vi "adsorption_rig_main-automation.vi"() -> ()   [LabVIEW 2024]
uses:
  adam5000_LLB/controls/adam-5000-serial-settings.ctl
  adam5000_LLB/controls/adam-5000-cmd-response.ctl
  adam5000_LLB/controls/state-enum.ctl
  adam5000_LLB/sub-vi/csv-file-logging/filepath-selection.ctl
  controls/sequence-states.ctl
  adam5000_LLB/controls/adam-5000-all-chassis-data.ctl
  adam5000_LLB/controls/adam-5000-all-module-datas.ctl
  adam5000_LLB/controls/digital-output-cluster.ctl
  adam5000_LLB/controls/digitial-input-cluster.ctl
  adam5000_LLB/controls/analog-output-cluster.ctl
  adam5000_LLB/controls/analog-input-cluster.ctl
  adam5000_LLB/controls/thermocouple-input-cluster.ctl
  adam5000_LLB/controls/adam-5000-chassis-cmd-ack.ctl
  adam5000_LLB/controls/adam-5000-chassis-module-types.ctl
  adam5000_LLB/controls/adam-5000-DO-user-input.ctl
  adam5000_LLB/controls/adam-5000-status-indicator-references.ctl
  controls/sequence-timings.ctl
  controls/state-indicator.ctl
panel:
  in  "Reset LD":bool
  out "longest delay":u32
  out "Next Log Event mS":u32
  in  "Tab Control":enum32{"System", "Settings"}(tab)
  out "Cycles Complete":u16
  out "sequence-state":T1
  out "pre":bool
  in  "Stop Sequence":bool
  in  "Start Sequence":bool
  out "Recirc":bool
  out "HR B":bool
  out "Ads 2":bool
  out "TC5":dbl
  out "TC1":dbl
  out "TC4":dbl
  in  "HR_B Time (s)":dbl
  in  "Ads_2 Time (s)":dbl
  in  "Isos_2 Time (s)":dbl
  out "Isos 2":bool
  out "HR A":bool
  out "Ads 1":bool
  out "TC12":dbl
  out "Isos 1":bool
  in  "# Cycles":u16=1
  in  "Recirc Time (s)":dbl
  in  "HR_A Time (s)":dbl
  in  "Ads_1 Time (s)":dbl
  in  "Isos_1 Time (s)":dbl
  in  "Flow 4":dbl
  in  "Flow 3":dbl
  in  "Flow 2":dbl
  in  "Flow 1":dbl
  in  "V9: EP1":bool
  in  "V12: EP4":bool
  in  "V10: EP2":bool
  in  "V11: EP3":bool
  in  "V15: \nRecirculation":bool
  in  "V14: HR2":bool
  out "TC9":dbl
  in  "V13: HR1":bool
  out "TC8":dbl
  in  "V8: In4":bool
  out "TC2":dbl
  out "TC3":dbl
  out "TC6":dbl
  out "TC7":dbl
  out "TC10":dbl
  out "TC11":dbl
  in  "V1: Ex1":bool
  in  "V2: Ex2":bool
  in  "V4: Ex4":bool
  in  "V5: In1":bool
  in  "V6: In2":bool
  in  "V7: In3":bool
  out "P1: Condenser":dbl
  out "P2: Adsorber 2":dbl
  out "P3: Adsorber 1":dbl
  out "P4: Evaporator":dbl
  in  "V3: Ex3":bool
  in  "Additional CSV Data Heading":string="Flow1,Flow2,Flow3,Flow4"
  in  "Chassis Settings":T2={"VISA resource name"="COM4", "baud rate (19200)"=19200, "Chassis ID"=1}
  in  "Log Filepath Selection":T3={"Log Filepath Source"=enum."Application Relative (Auto)", "Log File Path (Manual)"=path "C:/Users/iwheard/Documents/0000-labview/adam5000-generic-controller/data", "Log File Folder Name"="data", "log file name"="log", "Include Date in Filename"=TRUE, "Include Time in Filename"=TRUE}
  out "Log Filepath":path
  out "log start time":u32
  out "log-elapsed time":dbl format="%.2f"
  in  "CSV Data Headings":string="time (s),T1,T2,T3,T4,T5,T6,T7,T8,T9,T10,T11,T12,P1,P2,P3,P4, state"
  out "Logged Data String":string
  out "error":errorcluster
  out "Hz":dbl format="%_3g"
  in  "Sample Rate (Hz)":dbl=1.0 min=0.0001 max=4.0 format="%#_4g"
  out "File Open":bool
  out "Logging Active":bool
  out "Error Detected":bool
  in  "Reset":bool
  out "ADAM Connected":bool
  in  "Stop ADAM":bool
  in  "Start Logging":bool
  out "Program State":T4
  in  "Start ADAM":bool
  out "cmd-response":T6
  out "Status Indicators":T7
  in  "Debug Mode":bool
  out "Loop Time (mS)":u32
  out "Loop Counter":i32
  in  "exit":bool
  # "Adsorption Rig 2026"
  # "Built By: \nImogen Heard"
  # "Cold"
  # "Ambient"
  # "Hot"
  # "Pressure Sensors"
  # "NV-002"
  # "NV-001"
  # "NV-004"
  # "Flow 4"
  # "Flow 1"
  # "Flow 2"
  # "Sequence"
  # "NV-003"
  # "Flow 3"
  # "Condenser"
  # "Adsorber 1"
  # "Adsorber 2"
  # "Evaporator"
  # "Flow Meter Inputs"
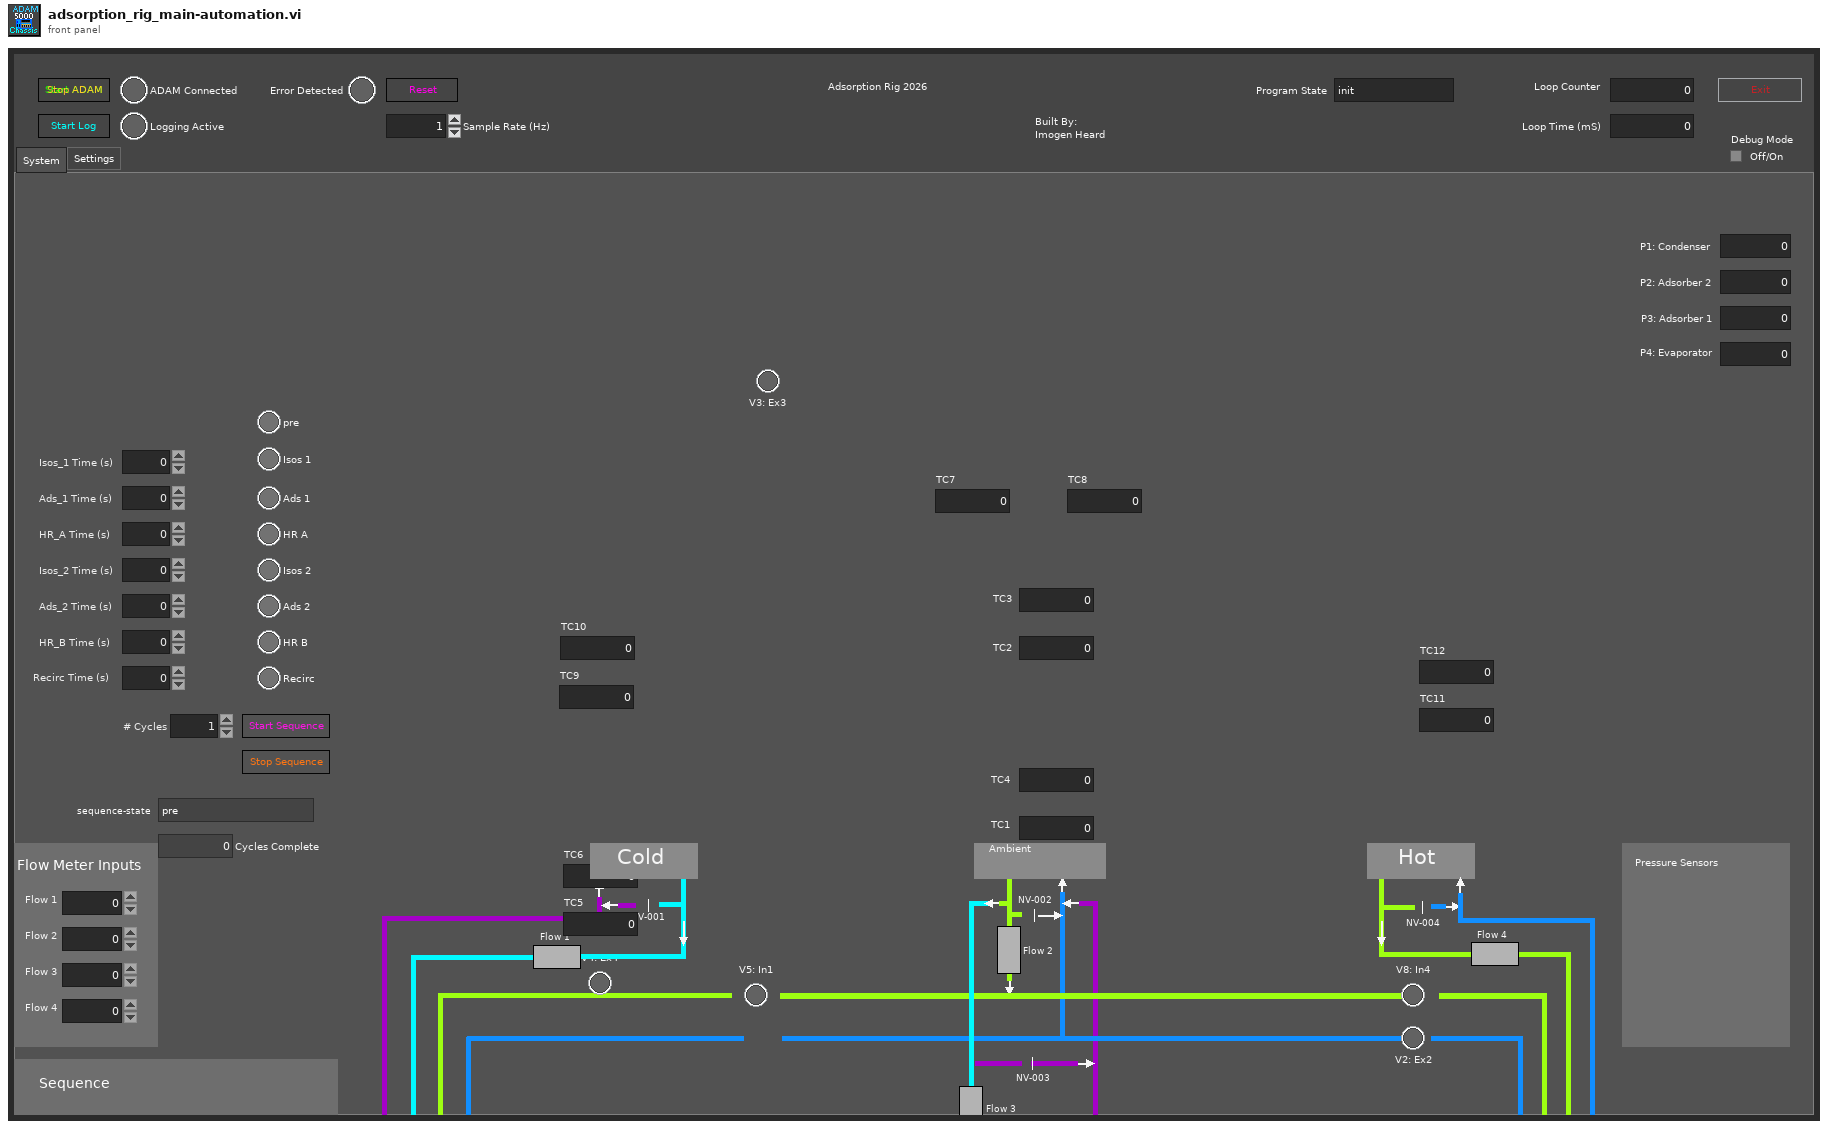
[diagram p1: front panel]
types:
  T1 = typedef "sequence-states.ctl" = enum16{"pre", "isos-1", "ads-1", "hr-a", "isos-2", "ads-2", "hr-b", "recirc", "cycle", "end"}
  T2 = typedef "adam-5000-serial-settings.ctl" = cluster{"VISA resource name":refnum<visa-resource-name>, "baud rate (19200)":u32, "Chassis ID":u8}
  T3 = typedef "filepath-selection.ctl" = cluster{"Log Filepath Source":enum16{"Application Relative (Auto)", "VI Relative (Auto)", "Complete Path (Manual)"}, "Log File Path (Manual)":path, "Log File Folder Name":string, "log file name":string, "Include Date in Filename":bool, "Include Time in Filename":bool}
  T4 = typedef "state-enum.ctl" = enum16{"init", "wait", "manual", "start", "run", "start-sequence", "stop-sequence", "sequence", "reset", "stop", "exit"}
  T5 = typedef "adam-5000-cmd-response.ctl" = cluster{"cmd string":string, "response":string}
  T6 = cluster{"cmd-response:0":T5, "cmd-response:1":T5, "cmd-response:2":T5, "cmd-response:3":T5, "cmd-response:4":T5, "cmd-response:5":T5, "cmd-response:6":T5, "cmd-response:7":T5}
  T7 = cluster{"status-indicator:0":cluster{"Sampling":bool, "Ack":bool}, "status-indicator:1":cluster{"Sampling":bool, "Ack":bool}, "status-indicator:2":cluster{"Sampling":bool, "Ack":bool}, "status-indicator:3":cluster{"Sampling":bool, "Ack":bool}, "status-indicator:4":cluster{"Sampling":bool, "Ack":bool}, "status-indicator:5":cluster{"Sampling":bool, "Ack":bool}, "status-indicator:6":cluster{"Sampling":bool, "Ack":bool}, "status-indicator:7":cluster{"Sampling":bool, "Ack":bool}}
  T8 = enum16{"Digital Output", "Digital Input", "Analog Output", "Analog Input", "Thermocouple", "Power Relay", "empty"}
  T9 = typedef "adam-5000-chassis-module-types.ctl" = cluster{"Slot 0: Module Type":enum16{"Digital Output", "Digital Input", "Analog Output", "Analog Input", "Thermocouple", "Power Relay", "empty"}, "Slot 1: Module Type":enum16{"Digital Output", "Digital Input", "Analog Output", "Analog Input", "Thermocouple", "Power Relay", "empty"}, "Slot 2: Module Type":enum16{"Digital Output", "Digital Input", "Analog Output", "Analog Input", "Thermocouple", "Power Relay", "empty"}, "Slot 3: Module Type":enum16{"Digital Output", "Digital Input", "Analog Output", "Analog Input", "Thermocouple", "Power Relay", "empty"}, "Slot 4: Module Type":enum16{"Digital Output", "Digital Input", "Analog Output", "Analog Input", "Thermocouple", "Power Relay", "empty"}, "Slot 5: Module Type":enum16{"Digital Output", "Digital Input", "Analog Output", "Analog Input", "Thermocouple", "Power Relay", "empty"}, "Slot 6: Module Type":enum16{"Digital Output", "Digital Input", "Analog Output", "Analog Input", "Thermocouple", "Power Relay", "empty"}, "Slot 7: Module Type":enum16{"Digital Output", "Digital Input", "Analog Output", "Analog Input", "Thermocouple", "Power Relay", "empty"}}
  T10 = typedef "adam-5000-chassis-cmd-ack.ctl" = cluster{"cmd-response:0":T5, "cmd-response:1":T5, "cmd-response:2":T5, "cmd-response:3":T5, "cmd-response:4":T5, "cmd-response:5":T5, "cmd-response:6":T5, "cmd-response:7":T5}
  T11 = typedef "adam-5000-all-chassis-data.ctl" = cluster{"slot:0":T12, "slot:1":T12, "slot:2":T12, "slot:3":T12, "slot:4":T12, "slot:5":T12, "slot:6":T12, "slot:7":T12}
  T12 = typedef "adam-5000-all-module-datas.ctl" = cluster{"Digital Outputs":T13, "Digital Inputs":T14, "Analog Outputs":T15, "Analog Inputs":T16, "Thermocouple Inputs (degC)":T17}
  T13 = typedef "digital-output-cluster.ctl" = cluster{"DO0":bool, "DO1":bool, "DO2":bool, "DO3":bool, "DO4":bool, "DO5":bool, "DO6":bool, "DO7":bool}
  T14 = typedef "digitial-input-cluster.ctl" = cluster{"DI0":bool, "DI1":bool, "DI2":bool, "DI3":bool, "DI4":bool, "DI5":bool, "DI6":bool, "DI7":bool}
  T15 = typedef "analog-output-cluster.ctl" = cluster{"AO0":dbl, "AO1":dbl, "AO2":dbl, "AO3":dbl}
  T16 = typedef "analog-input-cluster.ctl" = cluster{"AI0":dbl, "AI1":dbl, "AI2":dbl, "AI3":dbl, "AI4":dbl, "AI5":dbl, "AI6":dbl, "AI7":dbl}
  T17 = typedef "thermocouple-input-cluster.ctl" = cluster{"TC0":dbl, "TC1":dbl, "TC2":dbl, "TC3":dbl, "TC4":dbl, "TC5":dbl, "TC6":dbl}
  T18 = enum8{"Enabled", "Disabled", "Disabled and Grayed Out"}
  T19 = typedef "sequence-timings.ctl" = cluster{"Isos_1 Time":dbl, "Ads_1 Time":dbl, "HR_A Time":dbl, "Isos_2 Time":dbl, "Ads_2 Time":dbl, "HR_B Time":dbl, "Recirc Time":dbl}
  T20 = typedef "state-indicator.ctl" = cluster{"pre":bool, "Isos 1":bool, "Ads 1":bool, "HR A ":bool, "Isos 2":bool, "Ads 2":bool, "HR B":bool, "Recirc":bool}
  T21 = typedef "adam-5000-status-indicator-references.ctl" = cluster{"status-indicator:0":refnum<vi>, "status-indicator:1":refnum<vi>, "status-indicator:2":refnum<vi>, "status-indicator:3":refnum<vi>, "status-indicator:4":refnum<vi>, "status-indicator:5":refnum<vi>, "status-indicator:6":refnum<vi>, "status-indicator:7":refnum<vi>}
  T22 = typedef "adam-5000-DO-user-input.ctl" = cluster{"0:Digital Outputs":T13, "1:Digital Outputs":T13, "2:Digital Outputs":T13, "3:Digital Outputs":T13, "4:Digital Outputs":T13, "5:Digital Outputs":T13, "6:Digital Outputs":T13, "7:Digital Outputs":T13}
  T23 = cluster{"V1: Ex1":bool, "V2: Ex2":bool, "V3: Ex3":bool, "V4: Ex4":bool, "V5: In1":bool, "V6: In2":bool, "V7: In3":bool, "V8: In4":bool}
  T24 = cluster{"V9: EP1":bool, "V10: EP2":bool, "V11: EP3":bool, "V12: EP4":bool, "V13: HR1":bool, "V14: HR2":bool, "V15: \nRecirculation":bool, "V9: EP1":bool}
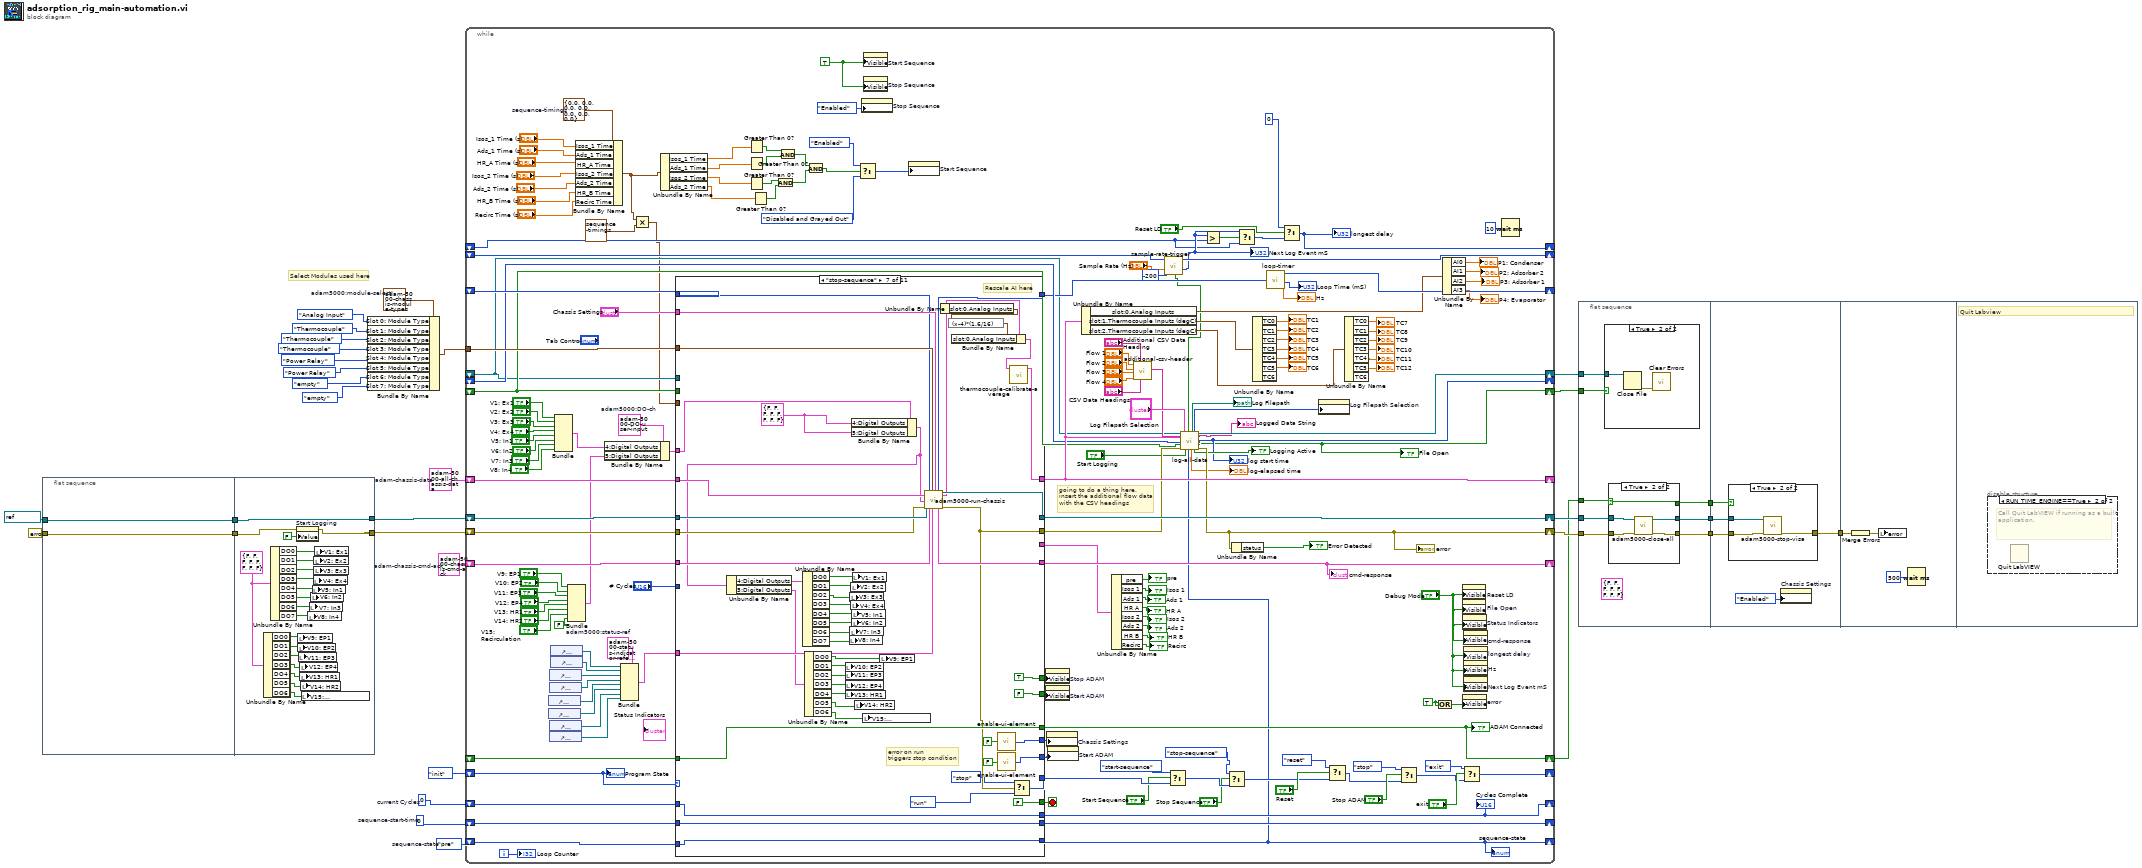
[diagram p0: block diagram]
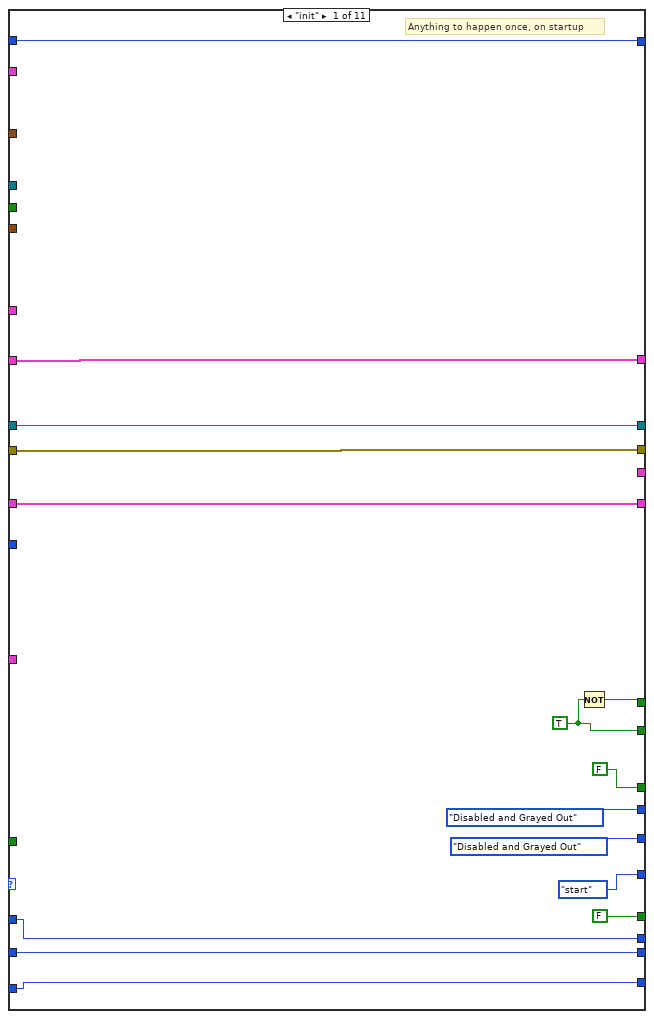
[diagram p6: hidden frame]
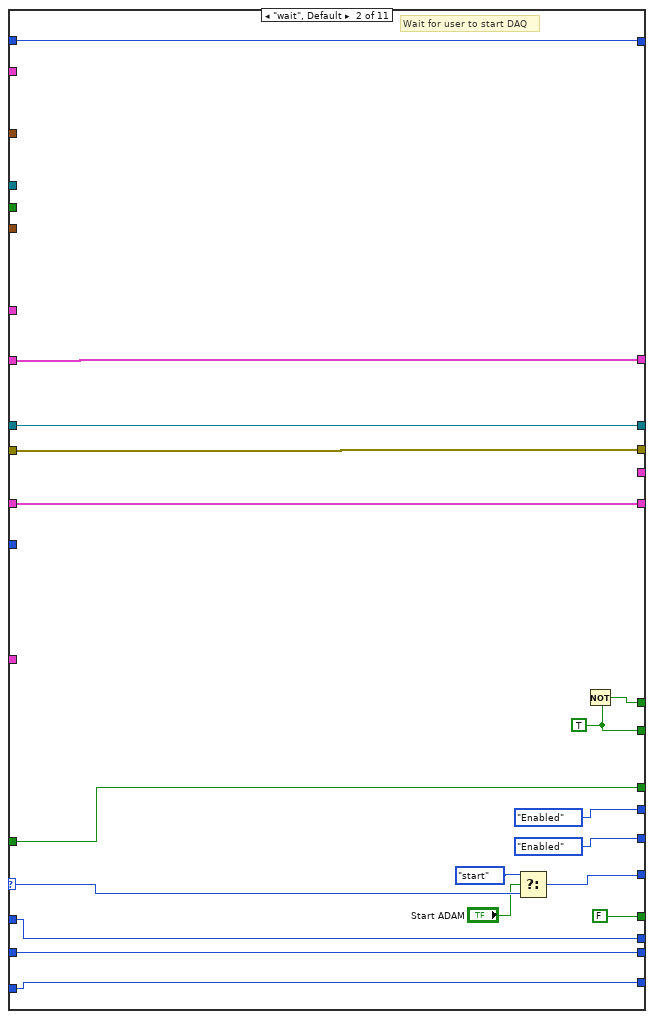
[diagram p7: hidden frame]
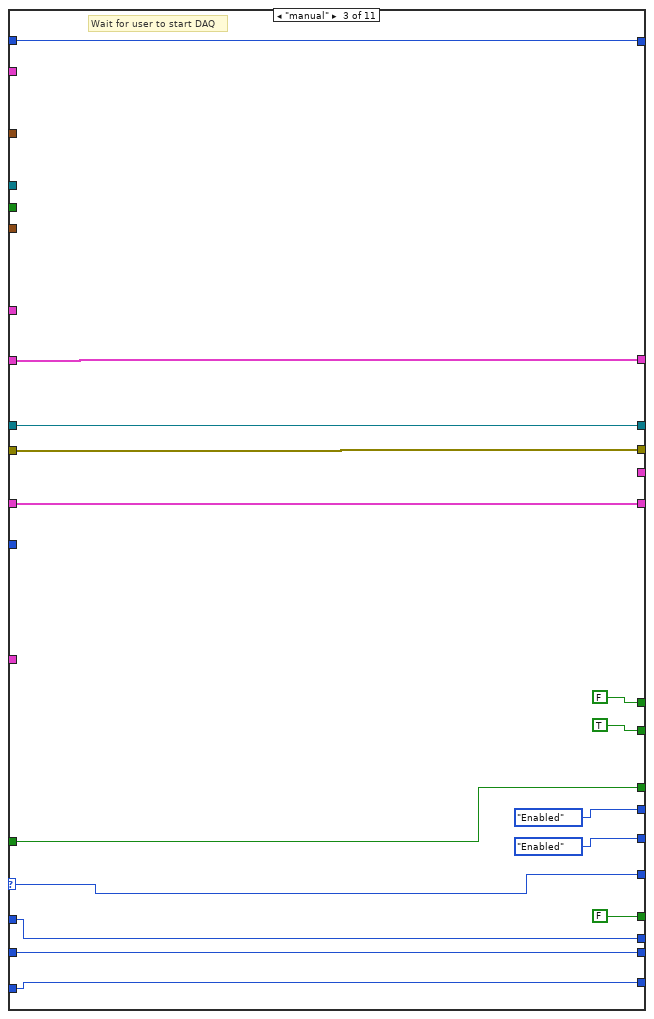
[diagram p8: hidden frame]
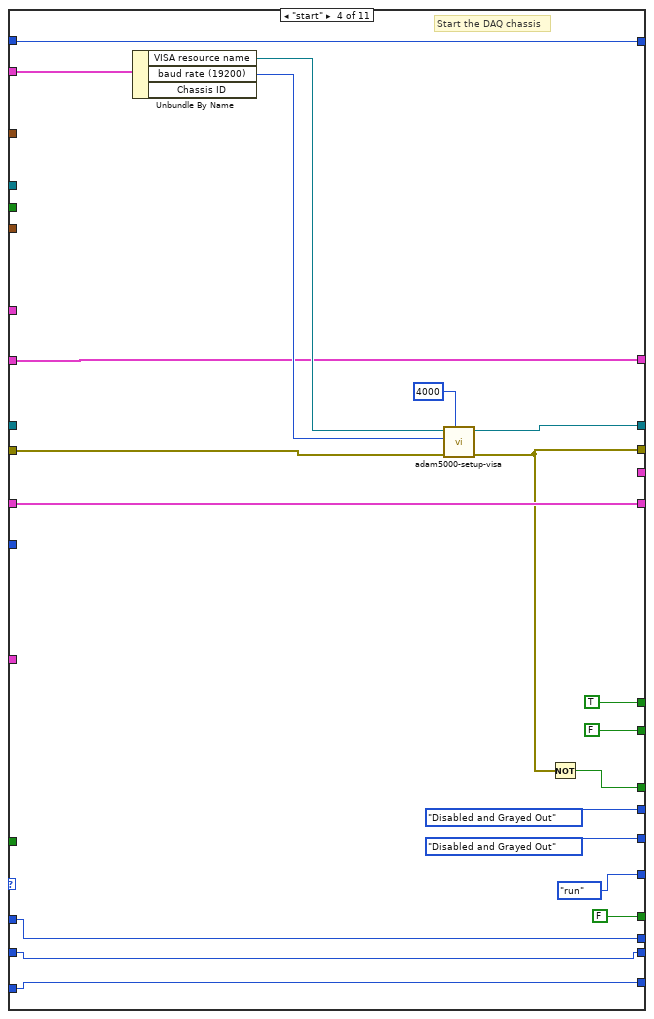
[diagram p9: hidden frame]
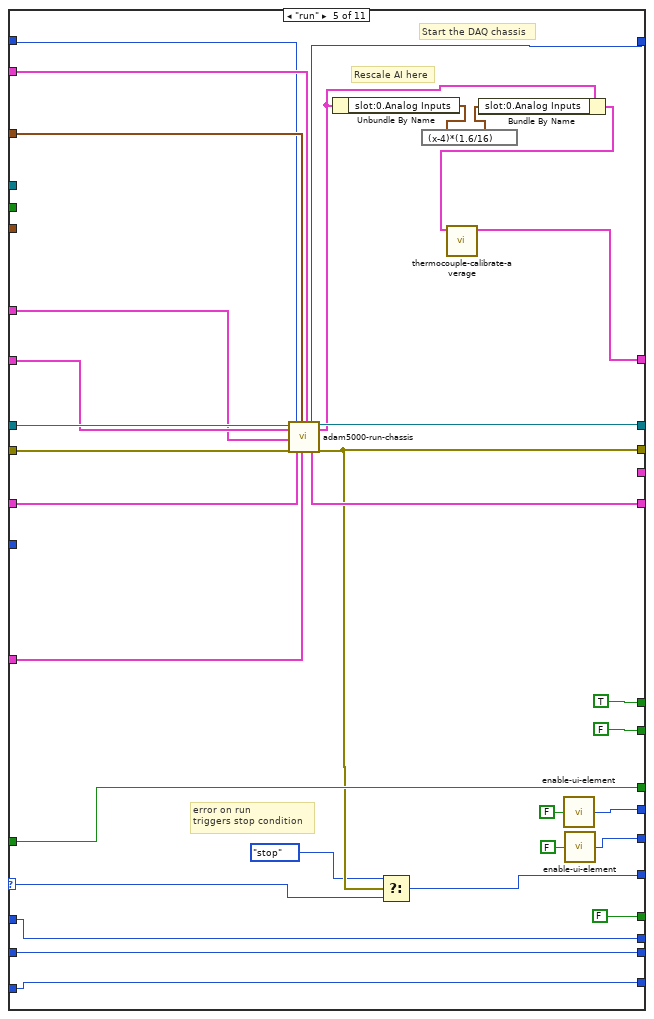
[diagram p10: hidden frame]
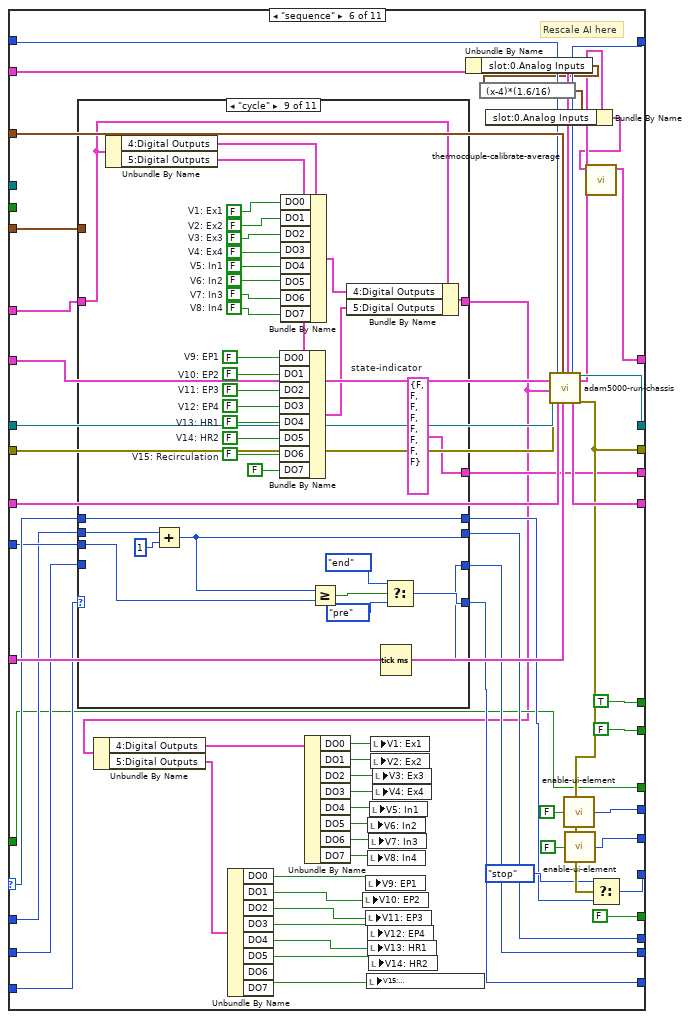
[diagram p11: hidden frame]
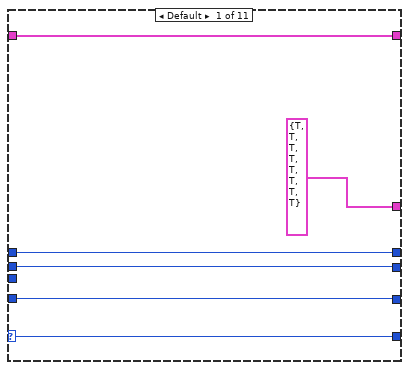
[diagram p12: hidden frame]
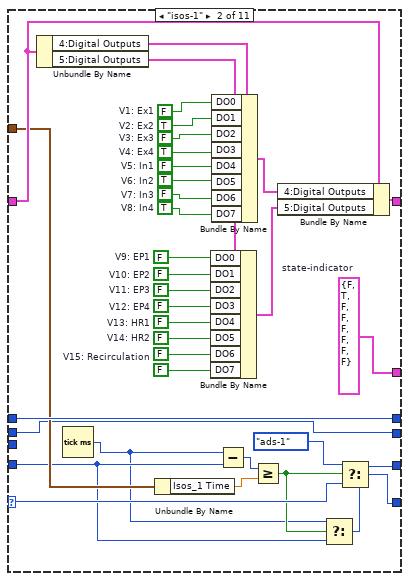
[diagram p13: hidden frame]
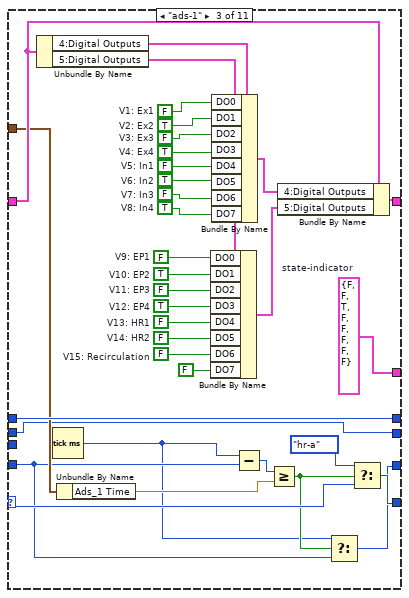
[diagram p14: hidden frame]
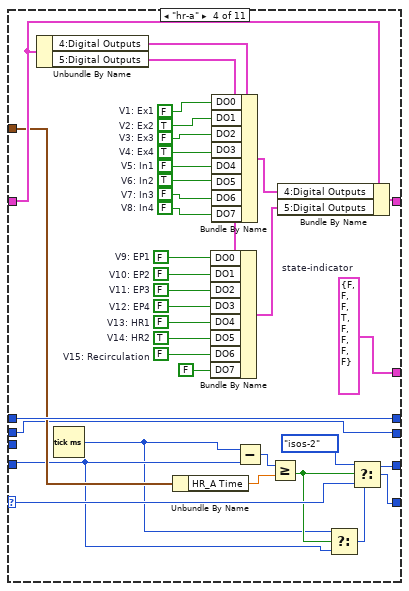
[diagram p15: hidden frame]
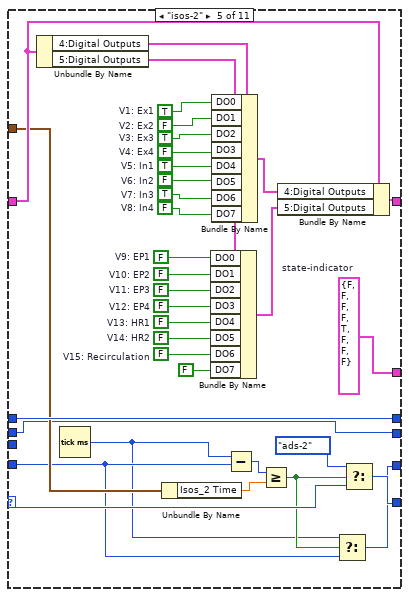
[diagram p16: hidden frame]
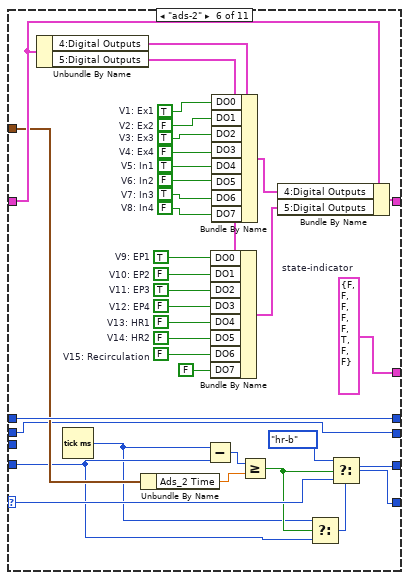
[diagram p17: hidden frame]
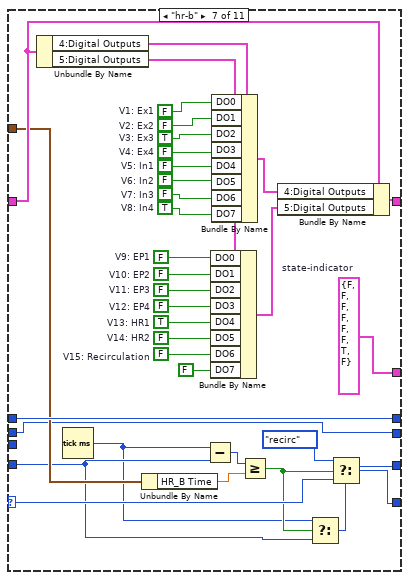
[diagram p18: hidden frame]
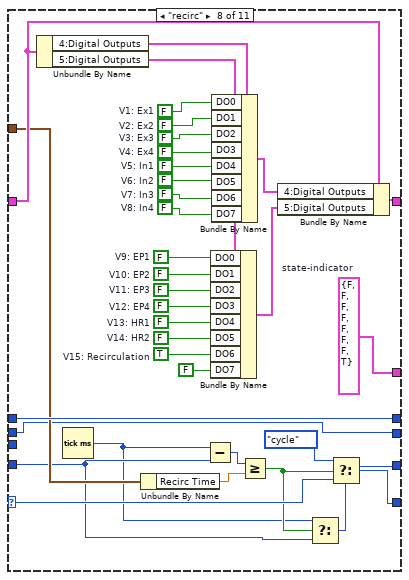
[diagram p19: hidden frame]
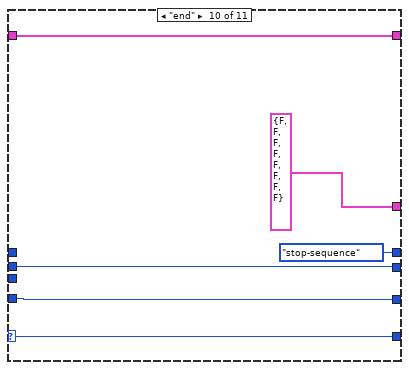
[diagram p20: hidden frame]
diagram:
  w1 = u16 0  # current Cycles
  w2 = u32 0  # sequence-start-time
  w3 = sequence-states."pre"  # sequence-state
  w23 = T9 {"Slot 0: Module Type"=enum."Digital Output", "Slot 1: Module Type"=enum."Digital Output", "Slot 2: Module Type"=enum."Digital Output", "Slot 3: Module Type"=enum."Digital Output", "Slot 4: Module Type"=enum."Digital Output", "Slot 5: Module Type"=enum."Digital Output", "Slot 6: Module Type"=enum."Digital Output", "Slot 7: Module Type"=enum."Digital Output"}  # adam5000:module-select
  w28 = T10 {"cmd-response:0"={"cmd string"="", "response"=""}, "cmd-response:1"={"cmd string"="", "response"=""}, "cmd-response:2"={"cmd string"="", "response"=""}, "cmd-response:3"={"cmd string"="", "response"=""}, "cmd-response:4"={"cmd string"="", "response"=""}, "cmd-response:5"={"cmd string"="", "response"=""}, "cmd-response:6"={"cmd string"="", "response"=""}, "cmd-response:7"={"cmd string"="", "response"=""}}  # adam-chassis-cmd-ack
  w29 = T11 {"slot:0"={"Digital Outputs"={"DO0"=FALSE, "DO1"=FALSE, "DO2"=FALSE, "DO3"=FALSE, "DO4"=FALSE, "DO5"=FALSE, "DO6"=FALSE, "DO7"=FALSE}, "Digital Inputs"={"DI0"=FALSE, "DI1"=FALSE, "DI2"=FALSE, "DI3"=FALSE, "DI4"=FALSE, "DI5"=FALSE, "DI6"=FALSE, "DI7"=FALSE}, "Analog Outputs"={"AO0"=0.0, "AO1"=0.0, "AO2"=0.0, "AO3"=0.0}, "Analog Inputs"={"AI0"=0.0, "AI1"=0.0, "AI2"=0.0, "AI3"=0.0, "AI4"=0.0, "AI5"=0.0, "AI6"=0.0, "AI7"=0.0}, "Thermocouple Inputs (degC)"={"TC0"=0.0, "TC1"=0.0, "TC2"=0.0, "TC3"=0.0, "TC4"=0.0, "TC5"=0.0, "TC6"=0.0}}, "slot:1"={"Digital Outputs"={"DO0"=FALSE, "DO1"=FALSE, "DO2"=FALSE, "DO3"=FALSE, "DO4"=FALSE, "DO5"=FALSE, "DO6"=FALSE, "DO7"=FALSE}, "Digital Inputs"={"DI0"=FALSE, "DI1"=FALSE, "DI2"=FALSE, "DI3"=FALSE, "DI4"=FALSE, "DI5"=FALSE, "DI6"=FALSE, "DI7"=FALSE}, "Analog Outputs"={"AO0"=0.0, "AO1"=0.0, "AO2"=0.0, "AO3"=0.0}, "Analog Inputs"={"AI0"=0.0, "AI1"=0.0, "AI2"=0.0, "AI3"=0.0, "AI4"=0.0, "AI5"=0.0, "AI6"=0.0, "AI7"=0.0}, "Thermocouple Inputs (degC)"={"TC0"=0.0, "TC1"=0.0, "TC2"=0.0, "TC3"=0.0, "TC4"=0.0, "TC5"=0.0, "TC6"=0.0}}, "slot:2"={"Digital Outputs"={"DO0"=FALSE, "DO1"=FALSE, "DO2"=FALSE, "DO3"=FALSE, "DO4"=FALSE, "DO5"=FALSE, "DO6"=FALSE, "DO7"=FALSE}, "Digital Inputs"={"DI0"=FALSE, "DI1"=FALSE, "DI2"=FALSE, "DI3"=FALSE, "DI4"=FALSE, "DI5"=FALSE, "DI6"=FALSE, "DI7"=FALSE}, "Analog Outputs"={"AO0"=0.0, "AO1"=0.0, "AO2"=0.0, "AO3"=0.0}, "Analog Inputs"={"AI0"=0.0, "AI1"=0.0, "AI2"=0.0, "AI3"=0.0, "AI4"=0.0, "AI5"=0.0, "AI6"=0.0, "AI7"=0.0}, "Thermocouple Inputs (degC)"={"TC0"=0.0, "TC1"=0.0, "TC2"=0.0, "TC3"=0.0, "TC4"=0.0, "TC5"=0.0, "TC6"=0.0}}, "slot:3"={"Digital Outputs"={"DO0"=FALSE, "DO1"=FALSE, "DO2"=FALSE, "DO3"=FALSE, "DO4"=FALSE, "DO5"=FALSE, "DO6"=FALSE, "DO7"=FALSE}, "Digital Inputs"={"DI0"=FALSE, "DI1"=FALSE, "DI2"=FALSE, "DI3"=FALSE, "DI4"=FALSE, "DI5"=FALSE, "DI6"=FALSE, "DI7"=FALSE}, "Analog Outputs"={"AO0"=0.0, "AO1"=0.0, "AO2"=0.0, "AO3"=0.0}, "Analog Inputs"={"AI0"=0.0, "AI1"=0.0, "AI2"=0.0, "AI3"=0.0, "AI4"=0.0, "AI5"=0.0, "AI6"=0.0, "AI7"=0.0}, "Thermocouple Inputs (degC)"={"TC0"=0.0, "TC1"=0.0, "TC2"=0.0, "TC3"=0.0, "TC4"=0.0, "TC5"=0.0, "TC6"=0.0}}, "slot:4"={"Digital Outputs"={"DO0"=FALSE, "DO1"=FALSE, "DO2"=FALSE, "DO3"=FALSE, "DO4"=FALSE, "DO5"=FALSE, "DO6"=FALSE, "DO7"=FALSE}, "Digital Inputs"={"DI0"=FALSE, "DI1"=FALSE, "DI2"=FALSE, "DI3"=FALSE, "DI4"=FALSE, "DI5"=FALSE, "DI6"=FALSE, "DI7"=FALSE}, "Analog Outputs"={"AO0"=0.0, "AO1"=0.0, "AO2"=0.0, "AO3"=0.0}, "Analog Inputs"={"AI0"=0.0, "AI1"=0.0, "AI2"=0.0, "AI3"=0.0, "AI4"=0.0, "AI5"=0.0, "AI6"=0.0, "AI7"=0.0}, "Thermocouple Inputs (degC)"={"TC0"=0.0, "TC1"=0.0, "TC2"=0.0, "TC3"=0.0, "TC4"=0.0, "TC5"=0.0, "TC6"=0.0}}, "slot:5"={"Digital Outputs"={"DO0"=FALSE, "DO1"=FALSE, "DO2"=FALSE, "DO3"=FALSE, "DO4"=FALSE, "DO5"=FALSE, "DO6"=FALSE, "DO7"=FALSE}, "Digital Inputs"={"DI0"=FALSE, "DI1"=FALSE, "DI2"=FALSE, "DI3"=FALSE, "DI4"=FALSE, "DI5"=FALSE, "DI6"=FALSE, "DI7"=FALSE}, "Analog Outputs"={"AO0"=0.0, "AO1"=0.0, "AO2"=0.0, "AO3"=0.0}, "Analog Inputs"={"AI0"=0.0, "AI1"=0.0, "AI2"=0.0, "AI3"=0.0, "AI4"=0.0, "AI5"=0.0, "AI6"=0.0, "AI7"=0.0}, "Thermocouple Inputs (degC)"={"TC0"=0.0, "TC1"=0.0, "TC2"=0.0, "TC3"=0.0, "TC4"=0.0, "TC5"=0.0, "TC6"=0.0}}, "slot:6"={"Digital Outputs"={"DO0"=FALSE, "DO1"=FALSE, "DO2"=FALSE, "DO3"=FALSE, "DO4"=FALSE, "DO5"=FALSE, "DO6"=FALSE, "DO7"=FALSE}, "Digital Inputs"={"DI0"=FALSE, "DI1"=FALSE, "DI2"=FALSE, "DI3"=FALSE, "DI4"=FALSE, "DI5"=FALSE, "DI6"=FALSE, "DI7"=FALSE}, "Analog Outputs"={"AO0"=0.0, "AO1"=0.0, "AO2"=0.0, "AO3"=0.0}, "Analog Inputs"={"AI0"=0.0, "AI1"=0.0, "AI2"=0.0, "AI3"=0.0, "AI4"=0.0, "AI5"=0.0, "AI6"=0.0, "AI7"=0.0}, "Thermocouple Inputs (degC)"={"TC0"=0.0, "TC1"=0.0, "TC2"=0.0, "TC3"=0.0, "TC4"=0.0, "TC5"=0.0, "TC6"=0.0}}, "slot:7"={"Digital Outputs"={"DO0"=FALSE, "DO1"=FALSE, "DO2"=FALSE, "DO3"=FALSE, "DO4"=FALSE, "DO5"=FALSE, "DO6"=FALSE, "DO7"=FALSE}, "Digital Inputs"={"DI0"=FALSE, "DI1"=FALSE, "DI2"=FALSE, "DI3"=FALSE, "DI4"=FALSE, "DI5"=FALSE, "DI6"=FALSE, "DI7"=FALSE}, "Analog Outputs"={"AO0"=0.0, "AO1"=0.0, "AO2"=0.0, "AO3"=0.0}, "Analog Inputs"={"AI0"=0.0, "AI1"=0.0, "AI2"=0.0, "AI3"=0.0, "AI4"=0.0, "AI5"=0.0, "AI6"=0.0, "AI7"=0.0}, "Thermocouple Inputs (degC)"={"TC0"=0.0, "TC1"=0.0, "TC2"=0.0, "TC3"=0.0, "TC4"=0.0, "TC5"=0.0, "TC6"=0.0}}}  # adam-chassis-data
  # "Select Modules used here"
  n1 = flat-sequence {
    tunnel: errorcluster {"status"=FALSE, "code"=0, "source"=""} ("error in") -> [w32]
    tunnel: refnum<visa-resource-name> "COM8" ("VISA Refnum out") -> [w33]
    tunnel: [w33] -> w5
    tunnel: [w32] -> w4
    tunnel: [w52] -> w12
    tunnel: [w50] -> w10
    tunnel: w5 -> [w52]
    tunnel: w4 -> [w51]
    frame #0 {
    }
    frame #1 {
      w41 = T13 {"DO0"=FALSE, "DO1"=FALSE, "DO2"=FALSE, "DO3"=FALSE, "DO4"=FALSE, "DO5"=FALSE, "DO6"=FALSE, "DO7"=FALSE} ("5:Digital Outputs")
      n2 = Unbundle By Name(w41) -> ("DO0"=w40:bool, "DO1"=w39:bool, "DO2"=w38:bool, "DO3"=w37:bool, "DO4"=w36:bool, "DO5"=w35:bool, "DO6"=w34:bool)
      n3 = Unbundle By Name(w41) -> ("DO0"=w49:bool, "DO1"=w48:bool, "DO2"=w47:bool, "DO3"=w46:bool, "DO4"=w45:bool, "DO5"=w44:bool, "DO6"=w43:bool, "DO7"=w42:bool)
      n4 = property on="Start Logging" class="Bool (strict)"(error in=w51, "Value"=FALSE ("Start Logging")) -> (error out=w50:errorcluster)  [unwired: 1 in, 1 out]
      n5 = local write "V9: EP1"(w40) -> ()
      n6 = local write "V10: EP2"(w39) -> ()
      n7 = local write "V11: EP3"(w38) -> ()
      n8 = local write "V12: EP4"(w37) -> ()
      n9 = local write "V13: HR1"(w36) -> ()
      n10 = local write "V14: HR2"(w35) -> ()
      n11 = local write "V15: \nRecirculation"(w34) -> ()
      n12 = local write "V8: In4"(w42) -> ()
      n13 = local write "V7: In3"(w43) -> ()
      n14 = local write "V6: In2"(w44) -> ()
      n15 = local write "V5: In1"(w45) -> ()
      n16 = local write "V4: Ex4"(w46) -> ()
      n17 = local write "V2: Ex2"(w48) -> ()
      n18 = local write "V3: Ex3"(w47) -> ()
      n19 = local write "V1: Ex1"(w49) -> ()
    }
  }
  n20 = Bundle By Name(cluster=w23, "Slot 0: Module Type"=T8."Analog Input", "Slot 1: Module Type"=T8."Thermocouple", "Slot 2: Module Type"=T8."Thermocouple" ("Slot 1: Module Type"), "Slot 3: Module Type"=T8."Thermocouple" ("Slot 1: Module Type"), "Slot 4: Module Type"=T8."Power Relay" ("Slot 1: Module Type"), "Slot 5: Module Type"=T8."Power Relay" ("Slot 1: Module Type"), "Slot 6: Module Type"=T8."empty" ("Slot 1: Module Type"), "Slot 7: Module Type"=T8."empty" ("Slot 1: Module Type")) -> (w14:T9)
  n21 = while {
    shift-right: [w201] -> _
    shift-left: state-enum."init" ("state-enum") -> [w185]
    shift-right: [w168] -> _
    shift-left: _ -> [w206]
    shift-right: [w193] -> w27
    shift-left: w12 -> [w209]
    shift-right: [w174] -> w26
    shift-left: w10 -> [w208]
    shift-right: [w176] -> _
    shift-left: w29 -> [w205]
    shift-right: [w187] -> _
    shift-left: w28 -> [w203]
    shift-right: [w191] -> w8
    shift-left: _ -> [w192]
    tunnel: w14 -> [w186]
    shift-right: [w164] -> w7
    shift-left: _ -> [w115]
    shift-right: [w165] -> _
    shift-left: _ -> [w175]
    shift-right: [w179] -> w6
    shift-left: _ -> [w114]
    shift-right: [w118] -> _
    shift-left: _ -> [w117]
    shift-right: [w106] -> _
    shift-left: _ -> [w110]
    shift-right: [w54] -> _
    shift-left: w3 -> [w103]
    shift-right: [w95] -> _
    shift-left: w2 -> [w94]
    shift-right: [w74] -> _
    shift-left: w1 -> [w75]
    i -> [w223]
    stop <- w194 stop-if-true
    w73 = TRUE ("Visible")
    w93 = T19 {"Isos_1 Time"=0.0, "Ads_1 Time"=0.0, "HR_A Time"=0.0, "Isos_2 Time"=0.0, "Ads_2 Time"=0.0, "HR_B Time"=0.0, "Recirc Time"=0.0}  # sequence-timings
    w212 = T21 {"status-indicator:0"=refnum, "status-indicator:1"=refnum, "status-indicator:2"=refnum, "status-indicator:3"=refnum, "status-indicator:4"=refnum, "status-indicator:5"=refnum, "status-indicator:6"=refnum, "status-indicator:7"=refnum}  # adam5000:status-ref
    w213 = T22 {"0:Digital Outputs"={"DO0"=FALSE, "DO1"=FALSE, "DO2"=FALSE, "DO3"=FALSE, "DO4"=FALSE, "DO5"=FALSE, "DO6"=FALSE, "DO7"=FALSE}, "1:Digital Outputs"={"DO0"=FALSE, "DO1"=FALSE, "DO2"=FALSE, "DO3"=FALSE, "DO4"=FALSE, "DO5"=FALSE, "DO6"=FALSE, "DO7"=FALSE}, "2:Digital Outputs"={"DO0"=FALSE, "DO1"=FALSE, "DO2"=FALSE, "DO3"=FALSE, "DO4"=FALSE, "DO5"=FALSE, "DO6"=FALSE, "DO7"=FALSE}, "3:Digital Outputs"={"DO0"=FALSE, "DO1"=FALSE, "DO2"=FALSE, "DO3"=FALSE, "DO4"=FALSE, "DO5"=FALSE, "DO6"=FALSE, "DO7"=FALSE}, "4:Digital Outputs"={"DO0"=FALSE, "DO1"=FALSE, "DO2"=FALSE, "DO3"=FALSE, "DO4"=FALSE, "DO5"=FALSE, "DO6"=FALSE, "DO7"=FALSE}, "5:Digital Outputs"={"DO0"=FALSE, "DO1"=FALSE, "DO2"=FALSE, "DO3"=FALSE, "DO4"=FALSE, "DO5"=FALSE, "DO6"=FALSE, "DO7"=FALSE}, "6:Digital Outputs"={"DO0"=FALSE, "DO1"=FALSE, "DO2"=FALSE, "DO3"=FALSE, "DO4"=FALSE, "DO5"=FALSE, "DO6"=FALSE, "DO7"=FALSE}, "7:Digital Outputs"={"DO0"=FALSE, "DO1"=FALSE, "DO2"=FALSE, "DO3"=FALSE, "DO4"=FALSE, "DO5"=FALSE, "DO6"=FALSE, "DO7"=FALSE}}  # adam5000:DO-ch
    w195 = TRUE ("Debug Mode")
    # "going to do a thing here,\ninsert the additional flow data \nwith the CSV headings"
    n22 = control-ref of="status-indicator:4"() -> (w217:refnum<vi>)
    n23 = control-ref of="status-indicator:5"() -> (w216:refnum<vi>)
    n24 = control-ref of="status-indicator:3"() -> (w218:refnum<vi>)
    n25 = control-ref of="status-indicator:6"() -> (w215:refnum<vi>)
    n26 = control-ref of="status-indicator:7"() -> (w214:refnum<vi>)
    n27 = control-ref of="status-indicator:2"() -> (w219:refnum<vi>)
    n28 = control-ref of="status-indicator:0"() -> (w221:refnum<vi>)
    n29 = control-ref of="status-indicator:1"() -> (w220:refnum<vi>)
    n30 = Bundle("V1: Ex1"="V1: Ex1", "V2: Ex2"="V2: Ex2", "V3: Ex3"="V3: Ex3", "V4: Ex4"="V4: Ex4", "V5: In1"="V5: In1", "V6: In2"="V6: In2", "V7: In3"="V7: In3", "V8: In4"="V8: In4") -> (w155:T23)  [unwired: 1 in]
    n31 = Bundle("V9: EP1"="V9: EP1", "V10: EP2"="V10: EP2", "V11: EP3"="V11: EP3", "V12: EP4"="V12: EP4", "V13: HR1"="V13: HR1", "V14: HR2"="V14: HR2", "V15: \nRecirculation"="V15: \nRecirculation", "V9: EP1"=FALSE) -> (w146:T24)  [unwired: 1 in]
    n32 = Bundle By Name(cluster=w93, "Isos_1 Time"="Isos_1 Time (s)", "Ads_1 Time"="Ads_1 Time (s)", "HR_A Time"="HR_A Time (s)", "Isos_2 Time"="Isos_2 Time (s)", "Ads_2 Time"="Ads_2 Time (s)", "HR_B Time"="HR_B Time (s)", "Recirc Time"="Recirc Time (s)") -> (w67:T19)
    n33 = Bundle By Name(cluster=w213, "4:Digital Outputs"=w155, "5:Digital Outputs"=w146) -> (w204:T22)
    n34 = Bundle(cluster=w212, "status-indicator:0"=w221, "status-indicator:1"=w220, "status-indicator:2"=w219, "status-indicator:3"=w218, "status-indicator:4"=w217, "status-indicator:5"=w216, "status-indicator:6"=w215, "status-indicator:7"=w214) -> (w202:T21)
    n35 = Multiply(x=w67, y=T19 {"Isos_1 Time"=1000.0, "Ads_1 Time"=1000.0, "HR_A Time"=1000.0, "Isos_2 Time"=1000.0, "Ads_2 Time"=1000.0, "HR_B Time"=1000.0, "Recirc Time"=1000.0}) -> (x*y=w65:T19)
    n36 = Unbundle By Name(w67) -> ("Isos_1 Time"=w71:dbl, "Ads_1 Time"=w70:dbl, "Isos_2 Time"=w69:dbl, "Ads_2 Time"=w68:dbl)
    n37 = case shown="\"stop-sequence\"" w185 {
      selector: w185 -> [_ w254 w267 _ w308 w351 _ _ _ _ _]
      tunnel: [state-enum."start" ("state-enum") w255 w267 state-enum."run" ("state-enum") w309 w368 w717 w747 state-enum."wait" ("state-enum") state-enum."wait" ("state-enum") state-enum."wait" ("state-enum")] -> w102
      tunnel: [T18."Disabled and Grayed Out" ("Disabled") T18."Enabled" ("Disabled") T18."Enabled" ("Disabled") T18."Disabled and Grayed Out" ("Disabled") w300 w360 w709 w742 T18."Disabled and Grayed Out" ("Disabled") T18."Disabled and Grayed Out" ("Disabled") T18."Enabled" ("Disabled")] -> w211
      tunnel: [T18."Disabled and Grayed Out" ("Disabled") T18."Enabled" ("Disabled") T18."Enabled" ("Disabled") T18."Disabled and Grayed Out" ("Disabled") w298 w358 w707 w740 T18."Disabled and Grayed Out" ("Disabled") T18."Disabled and Grayed Out" ("Disabled") T18."Enabled" ("Disabled")] -> w210
      tunnel: w209 -> [w235 w251 w269 _ w323 w380 w730 w738 w763 w794 w834]
      tunnel: [w235 w251 w269 w289 w321 w378 w728 w738 w757 w784 w822] -> w193
      tunnel: w208 -> [w234 w250 w268 w288 w322 w379 w729 w735 w762 w793 w833]
      tunnel: [w234 w250 w268 w278 w307 w367 w716 w735 w766 w783 w823] -> w173
      tunnel: "Chassis Settings" -> [_ _ _ w287 w320 w377 w727 _ _ w791 w831]
      tunnel: w186 -> [_ _ _ _ w319 w376 w726 _ w759 w792 w832]
      tunnel: w206 -> [w233 w248 w266 w282 w318 w375 w725 w736 w768 w785 w825]
      tunnel: [w233 w248 w266 w282 w317 w374 w724 w736 w768 w785 w825] -> w169
      tunnel: w205 -> [w232 w247 w265 w281 w316 w373 w723 w737 w761 w790 w830]
      tunnel: w204 -> [_ _ _ _ w315 w353 w700 _ _ _ _]
      tunnel: w203 -> [w231 w246 w264 w280 w314 w372 w722 w739 w767 w788 w828]
      tunnel: w202 -> [_ _ _ _ w313 w371 w721 _ _ w787 w827]
      tunnel: [w231 w246 w264 w280 w312 w370 w720 w739 w767 w786 w826] -> w187
      tunnel: [w232 w247 w265 w281 w296 w356 w705 w737 w760 w789 w829] -> w176
      tunnel: [FALSE FALSE FALSE FALSE FALSE FALSE FALSE FALSE FALSE FALSE TRUE] -> w194
      tunnel: [FALSE w244 w262 w277 w310 w342 w718 w748 FALSE FALSE FALSE] -> w191
      tunnel: w192 -> [_ w244 w262 _ w310 w342 w718 w748 _ w780 w820]
      tunnel: [w228 w242 TRUE ("Visible") FALSE ("Visible") FALSE ("Visible") FALSE ("Visible") FALSE ("Visible") FALSE ("Visible") FALSE ("Visible") TRUE ("Visible") w819] -> w184
      tunnel: [w227 w243 FALSE ("Visible") TRUE ("Visible") TRUE ("Visible") TRUE ("Visible") TRUE ("Visible") TRUE ("Visible") FALSE ("Visible") FALSE ("Visible") w819] -> w183
      tunnel: w115 -> [_ _ _ _ _ _ _ _ w754 _ w817]
      tunnel: w114 -> [_ _ _ _ _ _ _ _ w753 _ w818]
      tunnel: w103 -> [w226 w241 w259 w274 w294 w354 w703 _ w750 w777 w816]
      tunnel: [w226 w241 w259 w274 w294 w352 w703 sequence-states."pre" ("sequence-state") w750 w777 w816] -> w54
      tunnel: [w225 w240 w258 w273 w293 w346 w702 w733 w751 w776 w815] -> w95
      tunnel: w94 -> [w225 w240 w258 w273 w293 w349 w702 _ w751 w776 w815]
      tunnel: w65 -> [_ _ _ _ _ w348 _ _ _ _ _]
      tunnel: [_ _ _ _ _ w347 _ _ _ _ _] -> w78
      tunnel: "# Cycles" -> [_ _ _ _ _ w345 _ _ _ _ _]
      tunnel: w75 -> [w224 w239 w257 w272 w292 w344 w701 _ w752 w775 w814]
      tunnel: [w224 w239 w257 w272 w292 w343 w701 u16 0 ("current Cycles") w752 w775 w814] -> w74
      frame "init" {
        w228 = TRUE ("Visible")
        # "Anything to happen once, on startup"
        n38 = Not(x=w228) -> (.not. x?=w227:bool)
      }
      frame "wait", Default {
        w242 = TRUE ("Visible")
        # "Wait for user to start DAQ"
        n39 = Select(t=state-enum."start" ("state-enum"), s="Start ADAM", f=w254) -> (s? t:f=w255:T4)
        n40 = Not(x=w242) -> (.not. x?=w243:bool)
      }
      frame "manual" {
        # "Wait for user to start DAQ"
      }
      frame "start" {
        # "Start the DAQ chassis"
        n41 = Unbundle By Name(w287) -> ("VISA resource name"=w286:refnum<visa-resource-name>, "baud rate (19200)"=w285:u32)  [unwired: 1 out]
        n42 = call "adam5000-setup-visa.vi"("timeout (10sec)"=u32 4000, "error in"=w288, "baud rate (19200)"=w285, "VISA Refnum in"=w286) -> ("error out"=w278:errorcluster, "VISA Refnum out"=w289:refnum<visa-resource-name>)  [unwired: 6 in]
        n43 = Not(x=w278) -> (.not. x?=w277:bool)
      }
      frame "run" {
        # "Rescale AI here"
        # "error on run\ntriggers stop condition"
        # "Start the DAQ chassis"
        n44 = call "adam5000-run-chassis.vi"("VISA Refnum In"=w323, "adam-chassis-all-data-in"=w316, "adam-chassis-all-DO-in"=w315, "error in"=w322, "loop-time-in"=w318, "adam-chassis-cmd-response-in"=w314, "adam-chassis-module-select-in"=w319, "adam5000:status-ref-in"=w313, "Chassis Settings"=w320) -> ("loop-time-out"=w317:u32, "adam-chassis-cmd-response-out"=w312:T10, "VISA Refnum Out"=w321:refnum<visa-resource-name>, "adam-chassis-all-data-out"=w297:T11, "error out"=w307:errorcluster)  [unwired: 5 in, 1 out]
        n45 = Unbundle By Name(w297) -> ("slot:0.Analog Inputs"=w303:T16)
        n46 = Select(t=state-enum."stop", s=w307, f=w308) -> (s? t:f=w309:T4)
        n47 = expression code="(x-4)*(1.6/16)"(w303) -> (w302:T16)
        n48 = Bundle By Name(cluster=w297, "slot:0.Analog Inputs"=w302) -> (w295:T11)
        n49 = call "thermocouple-calibrate-average.vi"("adam-chassis-all-data-out in"=w295) -> ("adam-chassis-all-data-out out"=w296:T11)  [unwired: 10 in]
        n50 = call "enable-ui-element.vi"("Enable UI Element"=FALSE) -> ("UI Element State"=w300:T18)  [unwired: 8 in]
        n51 = call "enable-ui-element.vi"("Enable UI Element"=FALSE) -> ("UI Element State"=w298:T18)  [unwired: 8 in]
      }
      frame "sequence" {
        # "Rescale AI here"
        n52 = case shown="\"cycle\"" w354 {
          selector: w354 -> [w385 w395 w430 w465 w500 w535 w570 w605 _ w669 _]
          tunnel: w353 -> [w386 w419 w454 w489 w524 w559 w594 w629 w662 w667 w674]
          tunnel: [w386 w421 w456 w491 w526 w561 w596 w631 w664 w667 w672] -> w341
          tunnel: [w385 w394 w429 w464 w499 w534 w569 w604 w641 w669 sequence-states."isos-1" ("sequence-state")] -> w352
          tunnel: [w384 w415 w450 w485 w520 w555 w590 w625 w658 state-enum."stop-sequence" ("state-enum") w677] -> w350
          tunnel: w351 -> [w384 w415 w450 w485 w520 w555 w590 w625 w658 _ w677]
          tunnel: w349 -> [w383 w391 w424 w460 w495 w531 w566 w601 _ w666 w678]
          tunnel: w348 -> [_ w398 w433 w468 w503 w538 w573 w608 _ _ _]
          tunnel: [T20 {"pre"=TRUE, "Isos 1"=TRUE, "Ads 1"=TRUE, "HR A "=TRUE, "Isos 2"=TRUE, "Ads 2"=TRUE, "HR B"=TRUE, "Recirc"=TRUE} ("state-indicator") w392 w427 w462 w497 w532 w567 w602 w639 T20 {"pre"=FALSE, "Isos 1"=FALSE, "Ads 1"=FALSE, "HR A "=FALSE, "Isos 2"=FALSE, "Ads 2"=FALSE, "HR B"=FALSE, "Recirc"=FALSE} ("state-indicator") T20 {"pre"=TRUE, "Isos 1"=FALSE, "Ads 1"=FALSE, "HR A "=FALSE, "Isos 2"=FALSE, "Ads 2"=FALSE, "HR B"=FALSE, "Recirc"=FALSE} ("state-indicator")] -> w347
          tunnel: [w383 w388 w425 w458 w493 w530 w565 w600 w638 w666 w678] -> w346
          tunnel: w345 -> [_ _ _ _ _ _ _ _ w637 _ _]
          tunnel: w344 -> [w382 w387 w422 w457 w492 w527 w562 w597 w635 w670 w679]
          tunnel: [w382 w387 w422 w457 w492 w527 w562 w597 w632 w670 w679] -> w343
          frame Default {
          }
          frame "isos-1" {
            w392 = T20 {"pre"=FALSE, "Isos 1"=TRUE, "Ads 1"=FALSE, "HR A "=FALSE, "Isos 2"=FALSE, "Ads 2"=FALSE, "HR B"=FALSE, "Recirc"=FALSE}  # state-indicator
            w400 = FALSE  # V15: Recirculation
            w399 = FALSE  # V14: HR2
            w402 = FALSE  # V13: HR1
            w401 = FALSE  # V12: EP4
            w403 = FALSE  # V11: EP3
            w404 = FALSE  # V10: EP2
            w405 = FALSE  # V9: EP1
            w407 = TRUE  # V8: In4
            w408 = FALSE  # V7: In3
            w409 = TRUE  # V6: In2
            w410 = FALSE  # V5: In1
            w411 = TRUE  # V4: Ex4
            w412 = FALSE  # V3: Ex3
            w413 = TRUE  # V2: Ex2
            w414 = FALSE  # V1: Ex1
            n53 = Unbundle By Name(w419) -> ("4:Digital Outputs"=w418:T13, "5:Digital Outputs"=w416:T13)
            n54 = Tick Count (ms)() -> (millisecond timer value=w389:u32)
            n55 = Unbundle By Name(w398) -> ("Isos_1 Time"=w396:dbl)
            n56 = Bundle By Name(cluster=w416, "DO0"=w405, "DO1"=w404, "DO2"=w403, "DO3"=w401, "DO4"=w402, "DO5"=w399, "DO6"=w400, "DO7"=FALSE) -> (w417:T13)
            n57 = Bundle By Name(cluster=w418, "DO0"=w414, "DO1"=w413, "DO2"=w412, "DO3"=w411, "DO4"=w410, "DO5"=w409, "DO6"=w408, "DO7"=w407) -> (w420:T13)
            n58 = Subtract(x=w389, y=w391) -> (x-y=w397:u32)
            n59 = Greater Or Equal?(x=w397, y=w396) -> (x >= y?=w390:bool)
            n60 = Bundle By Name(cluster=w419, "4:Digital Outputs"=w420, "5:Digital Outputs"=w417) -> (w421:T22)
            n61 = Select(t=w389, s=w390, f=w391) -> (s? t:f=w388:u32)
            n62 = Select(t=sequence-states."ads-1", s=w390, f=w395) -> (s? t:f=w394:T1)
          }
          frame "ads-1" {
            w427 = T20 {"pre"=FALSE, "Isos 1"=FALSE, "Ads 1"=TRUE, "HR A "=FALSE, "Isos 2"=FALSE, "Ads 2"=FALSE, "HR B"=FALSE, "Recirc"=FALSE}  # state-indicator
            w435 = FALSE  # V15: Recirculation
            w434 = FALSE  # V14: HR2
            w437 = FALSE  # V13: HR1
            w436 = TRUE  # V12: EP4
            w438 = FALSE  # V11: EP3
            w439 = TRUE  # V10: EP2
            w440 = FALSE  # V9: EP1
            w442 = TRUE  # V8: In4
            w443 = FALSE  # V7: In3
            w444 = TRUE  # V6: In2
            w445 = FALSE  # V5: In1
            w446 = TRUE  # V4: Ex4
            w447 = FALSE  # V3: Ex3
            w448 = TRUE  # V2: Ex2
            w449 = FALSE  # V1: Ex1
            n63 = Unbundle By Name(w454) -> ("4:Digital Outputs"=w453:T13, "5:Digital Outputs"=w451:T13)
            n64 = Tick Count (ms)() -> (millisecond timer value=w423:u32)
            n65 = Unbundle By Name(w433) -> ("Ads_1 Time"=w431:dbl)
            n66 = Bundle By Name(cluster=w451, "DO0"=w440, "DO1"=w439, "DO2"=w438, "DO3"=w436, "DO4"=w437, "DO5"=w434, "DO6"=w435, "DO7"=FALSE) -> (w452:T13)
            n67 = Bundle By Name(cluster=w453, "DO0"=w449, "DO1"=w448, "DO2"=w447, "DO3"=w446, "DO4"=w445, "DO5"=w444, "DO6"=w443, "DO7"=w442) -> (w455:T13)
            n68 = Subtract(x=w423, y=w424) -> (x-y=w432:u32)
            n69 = Greater Or Equal?(x=w432, y=w431) -> (x >= y?=w426:bool)
            n70 = Bundle By Name(cluster=w454, "4:Digital Outputs"=w455, "5:Digital Outputs"=w452) -> (w456:T22)
            n71 = Select(t=w423, s=w426, f=w424) -> (s? t:f=w425:u32)
            n72 = Select(t=sequence-states."hr-a", s=w426, f=w430) -> (s? t:f=w429:T1)
          }
          frame "hr-a" {
            w462 = T20 {"pre"=FALSE, "Isos 1"=FALSE, "Ads 1"=FALSE, "HR A "=TRUE, "Isos 2"=FALSE, "Ads 2"=FALSE, "HR B"=FALSE, "Recirc"=FALSE}  # state-indicator
            w470 = FALSE  # V15: Recirculation
            w469 = TRUE  # V14: HR2
            w472 = FALSE  # V13: HR1
            w471 = FALSE  # V12: EP4
            w473 = FALSE  # V11: EP3
            w474 = FALSE  # V10: EP2
            w475 = FALSE  # V9: EP1
            w477 = FALSE  # V8: In4
            w478 = FALSE  # V7: In3
            w479 = TRUE  # V6: In2
            w480 = FALSE  # V5: In1
            w481 = TRUE  # V4: Ex4
            w482 = FALSE  # V3: Ex3
            w483 = TRUE  # V2: Ex2
            w484 = FALSE  # V1: Ex1
            n73 = Unbundle By Name(w489) -> ("4:Digital Outputs"=w488:T13, "5:Digital Outputs"=w486:T13)
            n74 = Tick Count (ms)() -> (millisecond timer value=w459:u32)
            n75 = Unbundle By Name(w468) -> ("HR_A Time"=w466:dbl)
            n76 = Bundle By Name(cluster=w486, "DO0"=w475, "DO1"=w474, "DO2"=w473, "DO3"=w471, "DO4"=w472, "DO5"=w469, "DO6"=w470, "DO7"=FALSE) -> (w487:T13)
            n77 = Bundle By Name(cluster=w488, "DO0"=w484, "DO1"=w483, "DO2"=w482, "DO3"=w481, "DO4"=w480, "DO5"=w479, "DO6"=w478, "DO7"=w477) -> (w490:T13)
            n78 = Subtract(x=w459, y=w460) -> (x-y=w467:u32)
            n79 = Greater Or Equal?(x=w467, y=w466) -> (x >= y?=w461:bool)
            n80 = Bundle By Name(cluster=w489, "4:Digital Outputs"=w490, "5:Digital Outputs"=w487) -> (w491:T22)
            n81 = Select(t=w459, s=w461, f=w460) -> (s? t:f=w458:u32)
            n82 = Select(t=sequence-states."isos-2", s=w461, f=w465) -> (s? t:f=w464:T1)
          }
          frame "isos-2" {
            w497 = T20 {"pre"=FALSE, "Isos 1"=FALSE, "Ads 1"=FALSE, "HR A "=FALSE, "Isos 2"=TRUE, "Ads 2"=FALSE, "HR B"=FALSE, "Recirc"=FALSE}  # state-indicator
            w505 = FALSE  # V15: Recirculation
            w504 = FALSE  # V14: HR2
            w507 = FALSE  # V13: HR1
            w506 = FALSE  # V12: EP4
            w508 = FALSE  # V11: EP3
            w509 = FALSE  # V10: EP2
            w510 = FALSE  # V9: EP1
            w512 = FALSE  # V8: In4
            w513 = TRUE  # V7: In3
            w514 = FALSE  # V6: In2
            w515 = TRUE  # V5: In1
            w516 = FALSE  # V4: Ex4
            w517 = TRUE  # V3: Ex3
            w518 = FALSE  # V2: Ex2
            w519 = TRUE  # V1: Ex1
            n83 = Unbundle By Name(w524) -> ("4:Digital Outputs"=w523:T13, "5:Digital Outputs"=w521:T13)
            n84 = Tick Count (ms)() -> (millisecond timer value=w494:u32)
            n85 = Unbundle By Name(w503) -> ("Isos_2 Time"=w501:dbl)
            n86 = Bundle By Name(cluster=w521, "DO0"=w510, "DO1"=w509, "DO2"=w508, "DO3"=w506, "DO4"=w507, "DO5"=w504, "DO6"=w505, "DO7"=FALSE) -> (w522:T13)
            n87 = Bundle By Name(cluster=w523, "DO0"=w519, "DO1"=w518, "DO2"=w517, "DO3"=w516, "DO4"=w515, "DO5"=w514, "DO6"=w513, "DO7"=w512) -> (w525:T13)
            n88 = Subtract(x=w494, y=w495) -> (x-y=w502:u32)
            n89 = Greater Or Equal?(x=w502, y=w501) -> (x >= y?=w496:bool)
            n90 = Bundle By Name(cluster=w524, "4:Digital Outputs"=w525, "5:Digital Outputs"=w522) -> (w526:T22)
            n91 = Select(t=w494, s=w496, f=w495) -> (s? t:f=w493:u32)
            n92 = Select(t=sequence-states."ads-2", s=w496, f=w500) -> (s? t:f=w499:T1)
          }
          frame "ads-2" {
            w532 = T20 {"pre"=FALSE, "Isos 1"=FALSE, "Ads 1"=FALSE, "HR A "=FALSE, "Isos 2"=FALSE, "Ads 2"=TRUE, "HR B"=FALSE, "Recirc"=FALSE}  # state-indicator
            w540 = FALSE  # V15: Recirculation
            w539 = FALSE  # V14: HR2
            w542 = FALSE  # V13: HR1
            w541 = FALSE  # V12: EP4
            w543 = TRUE  # V11: EP3
            w544 = FALSE  # V10: EP2
            w545 = TRUE  # V9: EP1
            w547 = FALSE  # V8: In4
            w548 = TRUE  # V7: In3
            w549 = FALSE  # V6: In2
            w550 = TRUE  # V5: In1
            w551 = FALSE  # V4: Ex4
            w552 = TRUE  # V3: Ex3
            w553 = FALSE  # V2: Ex2
            w554 = TRUE  # V1: Ex1
            n93 = Unbundle By Name(w559) -> ("4:Digital Outputs"=w558:T13, "5:Digital Outputs"=w556:T13)
            n94 = Tick Count (ms)() -> (millisecond timer value=w528:u32)
            n95 = Unbundle By Name(w538) -> ("Ads_2 Time"=w536:dbl)
            n96 = Subtract(x=w528, y=w531) -> (x-y=w537:u32)
            n97 = Bundle By Name(cluster=w556, "DO0"=w545, "DO1"=w544, "DO2"=w543, "DO3"=w541, "DO4"=w542, "DO5"=w539, "DO6"=w540, "DO7"=FALSE) -> (w557:T13)
            n98 = Bundle By Name(cluster=w558, "DO0"=w554, "DO1"=w553, "DO2"=w552, "DO3"=w551, "DO4"=w550, "DO5"=w549, "DO6"=w548, "DO7"=w547) -> (w560:T13)
            n99 = Greater Or Equal?(x=w537, y=w536) -> (x >= y?=w529:bool)
            n100 = Bundle By Name(cluster=w559, "4:Digital Outputs"=w560, "5:Digital Outputs"=w557) -> (w561:T22)
            n101 = Select(t=w528, s=w529, f=w531) -> (s? t:f=w530:u32)
            n102 = Select(t=sequence-states."hr-b", s=w529, f=w535) -> (s? t:f=w534:T1)
          }
          frame "hr-b" {
            w567 = T20 {"pre"=FALSE, "Isos 1"=FALSE, "Ads 1"=FALSE, "HR A "=FALSE, "Isos 2"=FALSE, "Ads 2"=FALSE, "HR B"=TRUE, "Recirc"=FALSE}  # state-indicator
            w575 = FALSE  # V15: Recirculation
            w574 = FALSE  # V14: HR2
            w577 = TRUE  # V13: HR1
            w576 = FALSE  # V12: EP4
            w578 = FALSE  # V11: EP3
            w579 = FALSE  # V10: EP2
            w580 = FALSE  # V9: EP1
            w582 = TRUE  # V8: In4
            w583 = FALSE  # V7: In3
            w584 = FALSE  # V6: In2
            w585 = FALSE  # V5: In1
            w586 = FALSE  # V4: Ex4
            w587 = TRUE  # V3: Ex3
            w588 = FALSE  # V2: Ex2
            w589 = FALSE  # V1: Ex1
            n103 = Unbundle By Name(w594) -> ("4:Digital Outputs"=w593:T13, "5:Digital Outputs"=w591:T13)
            n104 = Tick Count (ms)() -> (millisecond timer value=w563:u32)
            n105 = Unbundle By Name(w573) -> ("HR_B Time"=w571:dbl)
            n106 = Subtract(x=w563, y=w566) -> (x-y=w572:u32)
            n107 = Bundle By Name(cluster=w591, "DO0"=w580, "DO1"=w579, "DO2"=w578, "DO3"=w576, "DO4"=w577, "DO5"=w574, "DO6"=w575, "DO7"=FALSE) -> (w592:T13)
            n108 = Bundle By Name(cluster=w593, "DO0"=w589, "DO1"=w588, "DO2"=w587, "DO3"=w586, "DO4"=w585, "DO5"=w584, "DO6"=w583, "DO7"=w582) -> (w595:T13)
            n109 = Greater Or Equal?(x=w572, y=w571) -> (x >= y?=w564:bool)
            n110 = Bundle By Name(cluster=w594, "4:Digital Outputs"=w595, "5:Digital Outputs"=w592) -> (w596:T22)
            n111 = Select(t=w563, s=w564, f=w566) -> (s? t:f=w565:u32)
            n112 = Select(t=sequence-states."recirc", s=w564, f=w570) -> (s? t:f=w569:T1)
          }
          frame "recirc" {
            w602 = T20 {"pre"=FALSE, "Isos 1"=FALSE, "Ads 1"=FALSE, "HR A "=FALSE, "Isos 2"=FALSE, "Ads 2"=FALSE, "HR B"=FALSE, "Recirc"=TRUE}  # state-indicator
            w610 = TRUE  # V15: Recirculation
            w609 = FALSE  # V14: HR2
            w612 = FALSE  # V13: HR1
            w611 = FALSE  # V12: EP4
            w613 = FALSE  # V11: EP3
            w614 = FALSE  # V10: EP2
            w615 = FALSE  # V9: EP1
            w617 = FALSE  # V8: In4
            w618 = FALSE  # V7: In3
            w619 = FALSE  # V6: In2
            w620 = FALSE  # V5: In1
            w621 = FALSE  # V4: Ex4
            w622 = FALSE  # V3: Ex3
            w623 = FALSE  # V2: Ex2
            w624 = FALSE  # V1: Ex1
            n113 = Unbundle By Name(w629) -> ("4:Digital Outputs"=w628:T13, "5:Digital Outputs"=w626:T13)
            n114 = Tick Count (ms)() -> (millisecond timer value=w598:u32)
            n115 = Unbundle By Name(w608) -> ("Recirc Time"=w606:dbl)
            n116 = Subtract(x=w598, y=w601) -> (x-y=w607:u32)
            n117 = Bundle By Name(cluster=w626, "DO0"=w615, "DO1"=w614, "DO2"=w613, "DO3"=w611, "DO4"=w612, "DO5"=w609, "DO6"=w610, "DO7"=FALSE) -> (w627:T13)
            n118 = Bundle By Name(cluster=w628, "DO0"=w624, "DO1"=w623, "DO2"=w622, "DO3"=w621, "DO4"=w620, "DO5"=w619, "DO6"=w618, "DO7"=w617) -> (w630:T13)
            n119 = Greater Or Equal?(x=w607, y=w606) -> (x >= y?=w599:bool)
            n120 = Bundle By Name(cluster=w629, "4:Digital Outputs"=w630, "5:Digital Outputs"=w627) -> (w631:T22)
            n121 = Select(t=w598, s=w599, f=w601) -> (s? t:f=w600:u32)
            n122 = Select(t=sequence-states."cycle", s=w599, f=w605) -> (s? t:f=w604:T1)
          }
          frame "cycle" {
            w639 = T20 {"pre"=FALSE, "Isos 1"=FALSE, "Ads 1"=FALSE, "HR A "=FALSE, "Isos 2"=FALSE, "Ads 2"=FALSE, "HR B"=FALSE, "Recirc"=FALSE}  # state-indicator
            w643 = FALSE  # V15: Recirculation
            w642 = FALSE  # V14: HR2
            w645 = FALSE  # V13: HR1
            w644 = FALSE  # V12: EP4
            w646 = FALSE  # V11: EP3
            w647 = FALSE  # V10: EP2
            w648 = FALSE  # V9: EP1
            w650 = FALSE  # V8: In4
            w651 = FALSE  # V7: In3
            w652 = FALSE  # V6: In2
            w653 = FALSE  # V5: In1
            w654 = FALSE  # V4: Ex4
            w655 = FALSE  # V3: Ex3
            w656 = FALSE  # V2: Ex2
            w657 = FALSE  # V1: Ex1
            n123 = Unbundle By Name(w662) -> ("4:Digital Outputs"=w661:T13, "5:Digital Outputs"=w659:T13)
            n124 = Add(x=w635, y=u16 1) -> (x+y=w632:u16)
            n125 = Bundle By Name(cluster=w659, "DO0"=w648, "DO1"=w647, "DO2"=w646, "DO3"=w644, "DO4"=w645, "DO5"=w642, "DO6"=w643, "DO7"=FALSE) -> (w660:T13)
            n126 = Bundle By Name(cluster=w661, "DO0"=w657, "DO1"=w656, "DO2"=w655, "DO3"=w654, "DO4"=w653, "DO5"=w652, "DO6"=w651, "DO7"=w650) -> (w663:T13)
            n127 = Greater Or Equal?(x=w632, y=w637) -> (x >= y?=w636:bool)
            n128 = Bundle By Name(cluster=w662, "4:Digital Outputs"=w663, "5:Digital Outputs"=w660) -> (w664:T22)
            n129 = Tick Count (ms)() -> (millisecond timer value=w638:u32)
            n130 = Select(t=sequence-states."end", s=w636, f=sequence-states."pre") -> (s? t:f=w641:T1)
          }
          frame "end" {
          }
          frame "pre" {
            n131 = Bundle By Name(cluster=w674, "4:Digital Outputs"=T13 {"DO0"=FALSE, "DO1"=FALSE, "DO2"=FALSE, "DO3"=FALSE, "DO4"=FALSE, "DO5"=FALSE, "DO6"=FALSE, "DO7"=FALSE} ("0:Digital Outputs"), "5:Digital Outputs"=T13 {"DO0"=FALSE, "DO1"=FALSE, "DO2"=FALSE, "DO3"=FALSE, "DO4"=FALSE, "DO5"=FALSE, "DO6"=FALSE, "DO7"=FALSE}) -> (w672:T22)
          }
        }
        n132 = Unbundle By Name(w341) -> ("4:Digital Outputs"=w340:T13, "5:Digital Outputs"=w339:T13)
        n133 = Unbundle By Name(w339) -> ("DO0"=w330:bool, "DO1"=w329:bool, "DO2"=w328:bool, "DO3"=w327:bool, "DO4"=w326:bool, "DO5"=w325:bool, "DO6"=w324:bool)  [unwired: 1 out]
        n134 = Unbundle By Name(w340) -> ("DO0"=w338:bool, "DO1"=w337:bool, "DO2"=w336:bool, "DO3"=w335:bool, "DO4"=w334:bool, "DO5"=w333:bool, "DO6"=w332:bool, "DO7"=w331:bool)
        n135 = local write "V10: EP2"(w329) -> ()
        n136 = local write "V9: EP1"(w330) -> ()
        n137 = local write "V11: EP3"(w328) -> ()
        n138 = local write "V15: \nRecirculation"(w324) -> ()
        n139 = local write "V6: In2"(w333) -> ()
        n140 = local write "V8: In4"(w331) -> ()
        n141 = local write "V12: EP4"(w327) -> ()
        n142 = local write "V13: HR1"(w326) -> ()
        n143 = local write "V7: In3"(w332) -> ()
        n144 = local write "V14: HR2"(w325) -> ()
        n145 = local write "V5: In1"(w334) -> ()
        n146 = local write "V1: Ex1"(w338) -> ()
        n147 = local write "V2: Ex2"(w337) -> ()
        n148 = local write "V3: Ex3"(w336) -> ()
        n149 = local write "V4: Ex4"(w335) -> ()
        n150 = call "adam5000-run-chassis.vi"("VISA Refnum In"=w380, "adam-chassis-all-data-in"=w373, "adam-chassis-all-DO-in"=w341, "error in"=w379, "loop-time-in"=w375, "adam-chassis-cmd-response-in"=w372, "adam-chassis-module-select-in"=w376, "adam5000:status-ref-in"=w371, "Chassis Settings"=w377) -> ("loop-time-out"=w374:u32, "adam-chassis-cmd-response-out"=w370:T10, "VISA Refnum Out"=w378:refnum<visa-resource-name>, "adam-chassis-all-data-out"=w357:T11, "error out"=w367:errorcluster)  [unwired: 5 in, 1 out]
        n151 = Unbundle By Name(w357) -> ("slot:0.Analog Inputs"=w363:T16)
        n152 = expression code="(x-4)*(1.6/16)"(w363) -> (w362:T16)
        n153 = Bundle By Name(cluster=w357, "slot:0.Analog Inputs"=w362) -> (w355:T11)
        n154 = call "enable-ui-element.vi"("Enable UI Element"=FALSE) -> ("UI Element State"=w360:T18)  [unwired: 8 in]
        n155 = call "enable-ui-element.vi"("Enable UI Element"=FALSE) -> ("UI Element State"=w358:T18)  [unwired: 8 in]
        n156 = call "thermocouple-calibrate-average.vi"("adam-chassis-all-data-out in"=w355) -> ("adam-chassis-all-data-out out"=w356:T11)  [unwired: 10 in]
        n157 = Select(t=state-enum."stop", s=w367, f=w350) -> (s? t:f=w368:T4)
      }
      frame "stop-sequence" {
        w699 = T13 {"DO0"=FALSE, "DO1"=FALSE, "DO2"=FALSE, "DO3"=FALSE, "DO4"=FALSE, "DO5"=FALSE, "DO6"=FALSE, "DO7"=FALSE} ("4:Digital Outputs")
        # "Rescale AI here"
        # "error on run\ntriggers stop condition"
        n158 = Bundle By Name(cluster=w700, "4:Digital Outputs"=w699, "5:Digital Outputs"=w699) -> (w696:T22)
        n159 = Unbundle By Name(w696) -> ("4:Digital Outputs"=w698:T13, "5:Digital Outputs"=w697:T13)
        n160 = Unbundle By Name(w698) -> ("DO0"=w681:bool, "DO1"=w682:bool, "DO2"=w683:bool, "DO3"=w684:bool, "DO4"=w685:bool, "DO5"=w686:bool, "DO6"=w687:bool, "DO7"=w688:bool)
        n161 = Unbundle By Name(w697) -> ("DO0"=w695:bool, "DO1"=w694:bool, "DO2"=w693:bool, "DO3"=w692:bool, "DO4"=w691:bool, "DO5"=w690:bool, "DO6"=w689:bool)
        n162 = local write "V10: EP2"(w694) -> ()
        n163 = local write "V11: EP3"(w693) -> ()
        n164 = local write "V12: EP4"(w692) -> ()
        n165 = local write "V13: HR1"(w691) -> ()
        n166 = local write "V8: In4"(w688) -> ()
        n167 = local write "V3: Ex3"(w683) -> ()
        n168 = local write "V7: In3"(w687) -> ()
        n169 = local write "V4: Ex4"(w684) -> ()
        n170 = local write "V2: Ex2"(w682) -> ()
        n171 = local write "V5: In1"(w685) -> ()
        n172 = local write "V6: In2"(w686) -> ()
        n173 = local write "V1: Ex1"(w681) -> ()
        n174 = local write "V14: HR2"(w690) -> ()
        n175 = local write "V15: \nRecirculation"(w689) -> ()
        n176 = local write "V9: EP1"(w695) -> ()
        n177 = call "adam5000-run-chassis.vi"("VISA Refnum In"=w730, "adam-chassis-all-data-in"=w723, "adam-chassis-all-DO-in"=w696, "error in"=w729, "loop-time-in"=w725, "adam-chassis-cmd-response-in"=w722, "adam-chassis-module-select-in"=w726, "adam5000:status-ref-in"=w721, "Chassis Settings"=w727) -> ("loop-time-out"=w724:u32, "adam-chassis-cmd-response-out"=w720:T10, "VISA Refnum Out"=w728:refnum<visa-resource-name>, "adam-chassis-all-data-out"=w706:T11, "error out"=w716:errorcluster)  [unwired: 5 in, 1 out]
        n178 = Unbundle By Name(w706) -> ("slot:0.Analog Inputs"=w712:T16)
        n179 = expression code="(x-4)*(1.6/16)"(w712) -> (w711:T16)
        n180 = Bundle By Name(cluster=w706, "slot:0.Analog Inputs"=w711) -> (w704:T11)
        n181 = call "enable-ui-element.vi"("Enable UI Element"=FALSE) -> ("UI Element State"=w709:T18)  [unwired: 8 in]
        n182 = call "enable-ui-element.vi"("Enable UI Element"=FALSE) -> ("UI Element State"=w707:T18)  [unwired: 8 in]
        n183 = call "thermocouple-calibrate-average.vi"("adam-chassis-all-data-out in"=w704) -> ("adam-chassis-all-data-out out"=w705:T11)  [unwired: 10 in]
        n184 = Select(t=state-enum."stop", s=w716, f=state-enum."run") -> (s? t:f=w717:T4)
      }
      frame "start-sequence" {
        # "Rescale AI here"
        n185 = Tick Count (ms)() -> (millisecond timer value=w733:u32)
        n186 = call "enable-ui-element.vi"("Enable UI Element"=FALSE) -> ("UI Element State"=w742:T18)  [unwired: 8 in]
        n187 = call "enable-ui-element.vi"("Enable UI Element"=FALSE) -> ("UI Element State"=w740:T18)  [unwired: 8 in]
        n188 = Select(t=state-enum."stop", s=w735, f=state-enum."sequence") -> (s? t:f=w747:T4)
      }
      frame "reset" {
        # "Attempt to safe stop\nand clear errors"
        n189 = call "adam5000-close-all.vi"("VISA Refnum in"=w763, "adam5000:module-type-select"=w759, "adam5000:all-data-in"=w761, "error in (no error)"=w762) -> ("VISA Refnum out"=w757:refnum<visa-resource-name>, "adam5000:all-data-out"=w760:T11, "error out"=w764:errorcluster)  [unwired: 8 in, 1 out]
        n190 = case shown="True" w754 {
          tunnel: w753 -> [_ w774]
          frame False {
          }
          frame True {
            n191 = Close File(refnum=w774) -> (error out=w773:errorcluster)  [unwired: 1 in, 1 out]
            n192 = call <vilib>:"Clear Errors.vi"("error in (no error)"=w773) -> ()  [unwired: 5 in, 2 out]
          }
        }
        n193 = call "adam5000-stop-visa.vi"("error in (no error)"=w764, "VISA resource in"=w757) -> ("error out"=w758:errorcluster)  [unwired: 9 in]
        n194 = call <vilib>:"Clear Errors.vi"("error in (no error)"=w758) -> ("error out"=w766:errorcluster)  [unwired: 5 in, 1 out]
      }
      frame "stop" {
        # "Start the DAQ chassis"
        n195 = case shown="False" w780 {
          tunnel: w794 -> [w799 w813]
          tunnel: w793 -> [w798 w812]
          tunnel: w792 -> [_ w811]
          tunnel: w791 -> [_ w810]
          tunnel: w790 -> [w801 w809]
          tunnel: [w801 w808] -> w789
          tunnel: w788 -> [w800 w807]
          tunnel: w787 -> [_ w806]
          tunnel: [w800 w805] -> w786
          tunnel: [w799 w804] -> w784
          tunnel: [w798 w802] -> w783
          frame False {
          }
          frame True {
            n196 = call "adam5000-close-all.vi"("VISA Refnum in"=w813, "adam5000:module-type-select"=w811, "Chassis Settings in"=w810, "adam5000:all-data-in"=w809, "error in (no error)"=w812, "adam-chassis-cmd-ack"=w807, "adam5000:status-ref"=w806) -> ("VISA Refnum out"=w804:refnum<visa-resource-name>, "adam5000:all-data-out"=w808:T11, "adam-chassis-cmd-response-out"=w805:T10, "error out"=w803:errorcluster)  [unwired: 5 in]
            n197 = call "adam5000-stop-visa.vi"("error in (no error)"=w803, "VISA resource in"=w804) -> ("error out"=w802:errorcluster)  [unwired: 9 in]
          }
        }
      }
      frame "exit" {
        w819 = TRUE ("Visible")
        # "only performs\nshutdown if port\nis open"
        # "Start the DAQ chassis"
        n198 = case shown="True" w817 {
          tunnel: w818 -> [_ w838]
          frame False {
          }
          frame True {
            n199 = Close File(refnum=w838) -> ()  [unwired: 1 in, 2 out]
          }
        }
        n200 = case shown="True" w820 {
          tunnel: w834 -> [w841 w854]
          tunnel: w833 -> [w840 w853]
          tunnel: w832 -> [_ w852]
          tunnel: w831 -> [_ w851]
          tunnel: w830 -> [w842 w850]
          tunnel: [w842 w849] -> w829
          tunnel: w828 -> [w839 w848]
          tunnel: w827 -> [_ w847]
          tunnel: [w839 w846] -> w826
          tunnel: [w840 w844] -> w823
          tunnel: [w841 w843] -> w822
          frame False {
          }
          frame True {
            n201 = call "adam5000-close-all.vi"("VISA Refnum in"=w854, "adam5000:module-type-select"=w852, "Chassis Settings in"=w851, "adam5000:all-data-in"=w850, "error in (no error)"=w853, "adam-chassis-cmd-ack"=w848, "adam5000:status-ref"=w847) -> ("VISA Refnum out"=w843:refnum<visa-resource-name>, "adam5000:all-data-out"=w849:T11, "adam-chassis-cmd-response-out"=w846:T10, "error out"=w845:errorcluster)  [unwired: 5 in]
            n202 = call "adam5000-stop-visa.vi"("error in (no error)"=w845, "VISA resource in"=w843) -> ("error out"=w844:errorcluster)  [unwired: 9 in]
          }
        }
      }
    }
    "cmd-response" <- w187
    "ADAM Connected" <- w191
    "sequence-state" <- w54
    "Cycles Complete" <- w74
    n203 = Greater Than 0?(x=w71) -> (x > 0?=w64:bool)
    n204 = Greater Than 0?(x=w70) -> (x > 0?=w63:bool)
    n205 = Greater Than 0?(x=w69) -> (x > 0?=w62:bool)
    n206 = Greater Than 0?(x=w68) -> (x > 0?=w61:bool)
    n207 = And(x=w62, y=w61) -> (x .and. y?=w59:bool)
    n208 = And(x=w64, y=w63) -> (x .and. y?=w60:bool)
    n209 = And(x=w60, y=w59) -> (x .and. y?=w58:bool)
    n210 = Select(t=T18."Enabled" ("Disabled"), s=w58, f=T18."Disabled and Grayed Out") -> (s? t:f=w55:T18)
    n211 = property on="Stop Sequence" class="Bool"("DisabledEnum"=T18."Enabled" ("Disabled")) -> ()  [unwired: 2 in, 2 out]
    n212 = property on="Start Sequence" class="Bool"("Visible"=w73) -> ()  [unwired: 2 in, 2 out]
    n213 = property on="Stop Sequence" class="Bool"("Visible"=w73) -> ()  [unwired: 2 in, 2 out]
    n214 = property on="Start Sequence" class="Bool"("DisabledEnum"=w55) -> ()  [unwired: 2 in, 2 out]
    n215 = property on="Stop ADAM" class="Bool"("Visible"=w183) -> ()  [unwired: 2 in, 2 out]
    n216 = property on="Start ADAM" class="Bool"("Visible"=w184) -> ()  [unwired: 2 in, 2 out]
    n217 = property on="Chassis Settings" class="Clust (strict)"("DisabledEnum"=w211) -> ()  [unwired: 2 in, 2 out]
    n218 = property on="Start ADAM" class="Bool"("DisabledEnum"=w210) -> ()  [unwired: 2 in, 2 out]
    n219 = Unbundle By Name(w176) -> ("slot:0.Analog Inputs"=w138:T16, "slot:1.Thermocouple Inputs (degC)"=w133:T17, "slot:2.Thermocouple Inputs (degC)"=w126:T17)
    n220 = Unbundle By Name(w78) -> ("pre"=→"pre":bool, "Isos 1"=→"Isos 1":bool, "Ads 1"=→"Ads 1":bool, "HR A"=→"HR A":bool, "Isos 2"=→"Isos 2":bool, "Ads 2"=→"Ads 2":bool, "HR B"=→"HR B":bool, "Recirc"=→"Recirc":bool)
    n221 = call "additional-csv-header.vi"("CSV Data Headings"="CSV Data Headings", "Additional Text Heading"="Additional CSV Data Heading", "Flow 4"="Flow 4", "Flow 3"="Flow 3", "Flow 2"="Flow 2", "Flow 1"="Flow 1") -> ("new-csv-header"=w139:string)  [unwired: 5 in]
    n222 = call "sample-rate-trigger.vi"("last-event-mS in"=w117, "Sample Rate (Hz)"="Sample Rate (Hz)", "mS modifyer"=-200) -> ("triggered?"=w116:bool, "last-event-mS out"=w118:u32, "Elapsed Time mS"=w111:u32)  [unwired: 4 in, 1 out]
    "Next Log Event mS" <- w111
    n223 = Select(t=state-enum."start-sequence", s="Start Sequence", f=w102) -> (s? t:f=w101:T4)
    n224 = call "log-all-data.vi"("log-file-byte-stream"=w114, "CSV Data Headings"=w139, "adam5000:all-data-in"=w176, "log-start-time(mS)"=w175, "file open?"=w115, "error in (no error)"=w173, "Log Filepath Selection"="Log Filepath Selection", "Start Logging"="Start Logging", "Enable Log Trigger"=w116, "sequence-state"=w54) -> ("appended path for log file"=→"Log Filepath":path, "log-elapsed time"=→"log-elapsed time":dbl, "log-filepath-enable-state"=w178:T18, "Start Logging"=→"Logging Active":bool, "log-file-bytestream"=w179:refnum<file>, "Logged Data String"=→"Logged Data String":string, "log-start-time(mS)"=w165:u32, "file open?"=w164:bool, "error out"=w174:errorcluster)  [unwired: 1 in]
    "error" <- w174
    "File Open" <- w164
    "log start time" <- w165
    n225 = Greater?(x=w111, y=w110) -> (0:w112:bool)
    n226 = Select(t=state-enum."stop-sequence", s="Stop Sequence", f=w101) -> (s? t:f=w98:T4)
    n227 = Unbundle By Name(w174) -> ("status"=→"Error Detected":bool)
    n228 = Select(t=w111, s=w112, f=w110) -> (s? t:f=w109:u32)
    n229 = Unbundle By Name(w133) -> ("TC0"=→"TC1":dbl, "TC1"=→"TC2":dbl, "TC2"=→"TC3":dbl, "TC3"=→"TC4":dbl, "TC4"=→"TC5":dbl, "TC5"=→"TC6":dbl)  [unwired: 1 out]
    n230 = call "loop-timer.vi"("loop-time-in"=w169) -> ("Loop Time (mS)"=→"Loop Time (mS)":u32, "loop-time-out"=w168:u32, "Hz"=→"Hz":dbl)  [unwired: 8 in]
    n231 = Select(t=u32 0, s="Reset LD", f=w109) -> (s? t:f=w106:u32)
    "longest delay" <- w106
    n232 = property on="Log Filepath Selection" class="Clust (strict)"("DisabledEnum"=w178) -> ()  [unwired: 2 in, 2 out]
    n233 = Select(t=state-enum."reset", s="Reset", f=w98) -> (s? t:f=w189:T4)
    n234 = Unbundle By Name(w126) -> ("TC0"=→"TC7":dbl, "TC1"=→"TC8":dbl, "TC2"=→"TC9":dbl, "TC3"=→"TC10":dbl, "TC4"=→"TC11":dbl, "TC5"=→"TC12":dbl)  [unwired: 1 out]
    n235 = Select(t=state-enum."stop", s="Stop ADAM", f=w189) -> (s? t:f=w198:T4)
    n236 = Or(x=w195, y=w195) -> (x .or. y?=w222:bool)
    n237 = Unbundle By Name(w138) -> ("AI0"=→"P1: Condenser":dbl, "AI1"=→"P2: Adsorber 2":dbl, "AI2"=→"P3: Adsorber 1":dbl, "AI3"=→"P4: Evaporator":dbl)
    n238 = property on="Reset LD" class="Bool"("Visible"="Debug Mode") -> ()  [unwired: 2 in, 2 out]
    n239 = property on="File Open" class="Bool (strict)"("Visible"="Debug Mode") -> ()  [unwired: 2 in, 2 out]
    n240 = property on="Status Indicators" class="Clust (strict)"("Visible"="Debug Mode") -> ()  [unwired: 2 in, 2 out]
    n241 = property on="error" class="Clust (strict)"("Visible"=w222) -> ()  [unwired: 2 in, 2 out]
    n242 = Select(t=state-enum."exit", s="exit", f=w198) -> (s? t:f=w201:T4)
    n243 = property on="cmd-response" class="Clust (strict)"("Visible"="Debug Mode") -> ()  [unwired: 2 in, 2 out]
    n244 = property on="longest delay" class="DigNum (strict)"("Visible"="Debug Mode") -> ()  [unwired: 2 in, 2 out]
    n245 = property on="Hz" class="DigNum (strict)"("Visible"="Debug Mode") -> ()  [unwired: 2 in, 2 out]
    n246 = property on="Next Log Event mS" class="DigNum (strict)"("Visible"="Debug Mode") -> ()  [unwired: 2 in, 2 out]
    n247 = Wait (ms)(milliseconds to wait=u32 10) -> ()  [unwired: 1 out]
    "Loop Counter" <- w223
    "Program State" <- w185
  }
  n248 = flat-sequence {
    tunnel: w27 -> [w862]
    tunnel: w26 -> [w861]
    tunnel: [w860] -> w25
    tunnel: [w859] -> w24
    tunnel: w8 -> [w858]
    tunnel: [w857] -> w9
    tunnel: w7 -> [w856]
    tunnel: w6 -> [w855]
    tunnel: [w877] -> w30
    tunnel: w25 -> [w876]
    tunnel: w24 -> [w875]
    tunnel: w9 -> [w873]
    tunnel: w30 -> [w883]
    frame #0 {
      (unwired) T13 {"DO0"=FALSE, "DO1"=FALSE, "DO2"=FALSE, "DO3"=FALSE, "DO4"=FALSE, "DO5"=FALSE, "DO6"=FALSE, "DO7"=FALSE} ("5:Digital Outputs")
      n249 = case shown="True" w856 {
        tunnel: w855 -> [_ w864]
        frame False {
        }
        frame True {
          n250 = Close File(refnum=w864) -> (error out=w863:errorcluster)  [unwired: 1 in, 1 out]
          n251 = call <vilib>:"Clear Errors.vi"("error in (no error)"=w863) -> ()  [unwired: 5 in, 2 out]
        }
      }
      n252 = case shown="True" w858 {
        selector: w858 -> [w865 w868]
        tunnel: w862 -> [w867 w872]
        tunnel: w861 -> [w866 w871]
        tunnel: [w866 w870] -> w860
        tunnel: [w867 w869] -> w859
        tunnel: [w865 w868] -> w857
        frame False {
        }
        frame True {
          n253 = call "adam5000-close-all.vi"("VISA Refnum in"=w872, "error in (no error)"=w871) -> ("VISA Refnum out"=w869:refnum<visa-resource-name>, "error out"=w870:errorcluster)  [unwired: 10 in, 2 out]
        }
      }
    }
    frame #1 {
      n254 = case shown="True" w873 {
        tunnel: [w878 w881] -> w877
        tunnel: w876 -> [w878 w880]
        tunnel: w875 -> [_ w879]
        frame False {
        }
        frame True {
          n255 = call "adam5000-stop-visa.vi"("error in (no error)"=w880, "VISA resource in"=w879) -> ("error out"=w881:errorcluster)  [unwired: 9 in]
        }
      }
      n256 = property on="Chassis Settings" class="Clust (strict)"("DisabledEnum"=T18."Enabled" ("Disabled")) -> ()  [unwired: 2 in, 2 out]
    }
    frame #2 {
      n257 = Merge Errors(w883) -> (w882:errorcluster)
      n258 = local write "error"(w882) -> ()
      n259 = Wait (ms)(milliseconds to wait=u32 500) -> ()  [unwired: 1 out]
    }
    frame #3 {
      # "Quit Labview"
      n260 = disable-structure "Conditional Disable Structure" shown="RUN_TIME_ENGINE==True" {
        frame condition #0 (active) {
        }
        frame condition #1 {
          # "Call Quit LabVIEW if running as a built application."
          n261 = Quit LabVIEW() -> ()  [unwired: 1 in]
        }
      }
    }
  }
